vi "Certification Authority.vi"() -> ()   [LabVIEW 2013]
uses:
  certificate -- cluster.ctl
  certificate signature request (CA) -- cluster.ctl
  encryption key -- cluster.ctl
  initca -- cluster.ctl
  certificate signature request (Server) -- cluster.ctl
  <vilib>/Platform/browser.llb/Open URL in Default Browser (string).vi
  <vilib>/Platform/browser.llb/Open URL in Default Browser (path).vi
  <userlib>/_OpenG.lib/file/file.llb/Build Path - Traditional__ogtk.vi
  <userlib>/_OpenG.lib/file/file.llb/File Exists - Scalar__ogtk.vi
  <userlib>/_OpenG.lib/file/file.llb/Convert File Extension (String)__ogtk.vi
  Certification Authority.lvclass
panel:
  in  "Tab Control":T1(tab)
  in  "Root Certificate":path
  in  "Root Private Key":path
  in  "Open Certificates Folder":bool
  in  "Open GitHub Project Page":bool
  in  "Hosts":string[](array[string])=["lvtls-ca.example", "www.lvtls-ca.example"]
  in  "Common Name":string="lvtls-ca.example"
  in  "Generate Root Certificate":bool
  out "CFSSL App found":bool
  out "Root Certificate found":bool
  in  "Open Cloudflare Release Page":bool
  in  "Generate Server Certificates":bool
  in  "Servers":cluster{"hosts":string[], "name":string}[](array[cluster])
  out "Certificates":T2(array[cluster])
  in  "Certificates and Keys":i32(listbox)
  out "Selected Certificate":string
  # "ROOT (CERTIFICATE AUTHORITY)\nIf you have a root certificate and private key, import it to generate server certificate files.\nIf you don't have a root certificate, fill in the fields in section 2 and generate one."
  # "GENERATE ROOT CERTIFICATE\nIf you don't have a root certificate, fill in the fields below and generate one."
  # "3- SERVERS\nList each server you want to create certificates for."
  # "1- Give your server a unique \"Common Name\" in the name field\n2- List the hostnames that client can use to connect to this server\n     (this is not an IP address).\n3- Listing multiple servers will create certificates in batch mode.\n\n\nEx: \n\nname: myServerName\nhosts: localdomain.company.com; www.localdomain.company.com"
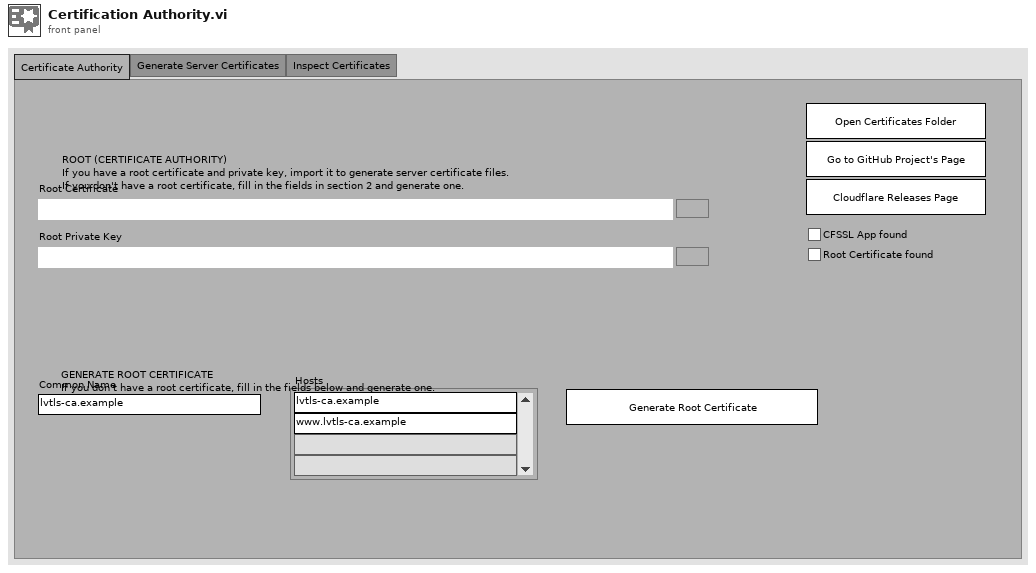
[diagram p1: front panel]
types:
  T1 = enum32{"Certificate Authority", "Generate Server Certificates", "Inspect Certificates"}
  T2 = cluster{"Type":string, "Decoded Certificate":string}[]
  T3 = enum32{"Invalid", "Standard", "Closed", "Hidden", "Minimized", "Maximized"}
  T4 = enum32{"invalid app kind", "Development System", "Run Time System", "Student Edition", "Embedded LabVIEW", "Evaluation", "Custom"}
  T5 = enum16{"open", "replace", "create", "open or create", "replace or create", "replace or create with confirmation"}
  T6 = typedef "Certification Authority.lvclass/certificate signature request (CA) -- cluster.ctl" = cluster{"CN":string, "hosts":string[], "key":T7, "ca":T8}
  T7 = typedef "Certification Authority.lvclass/encryption key -- cluster.ctl" = cluster{"algo":string, "size":u32}
  T8 = typedef "Certification Authority.lvclass/initca -- cluster.ctl" = cluster{"pathlen":u8, "expiry":string}
  T9 = typedef "Certification Authority.lvclass/certificate signature request (Server) -- cluster.ctl" = cluster{"CN":string, "hosts":string[], "key":T7}
  T10 = typedef "Certification Authority.lvclass/certificate -- cluster.ctl" = cluster{"cert":string, "csr":string, "key":string}
  T11 = cluster{"Core":cluster{"Current VI Reference":refnum<vi>, "Close Panel on Exit?":bool}, "CA":T10, "Server":T10, "cfssl path":path, "temp folder":path, "Certificates Folder":path, "Root name":string, "Root Certificate":path, "Root Private Key":path, "Active CN":string, "Active Hosts":string[], "next":i32, "Processing Queue":cluster{"hosts":string[], "name":string}[]}
  T12 = cluster{"Current VI Reference":refnum<vi>, "Close Panel on Exit?":bool}
  T13 = cluster{"Type":string, "Decoded String":string}[]
  T14 = enum8{"Enabled", "Disabled", "Disabled and Grayed Out"}
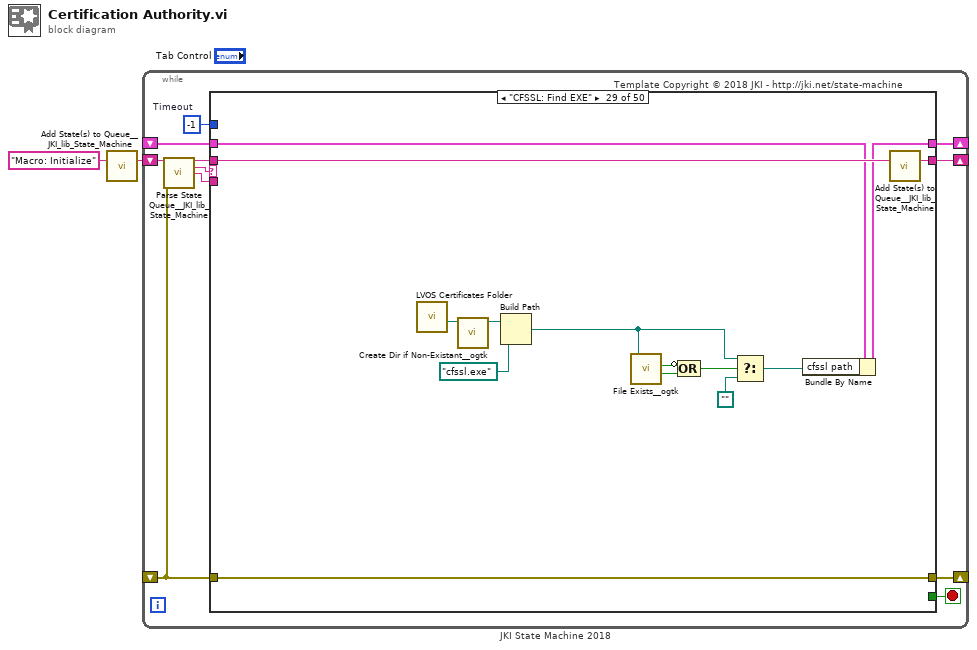
[diagram p0: block diagram]
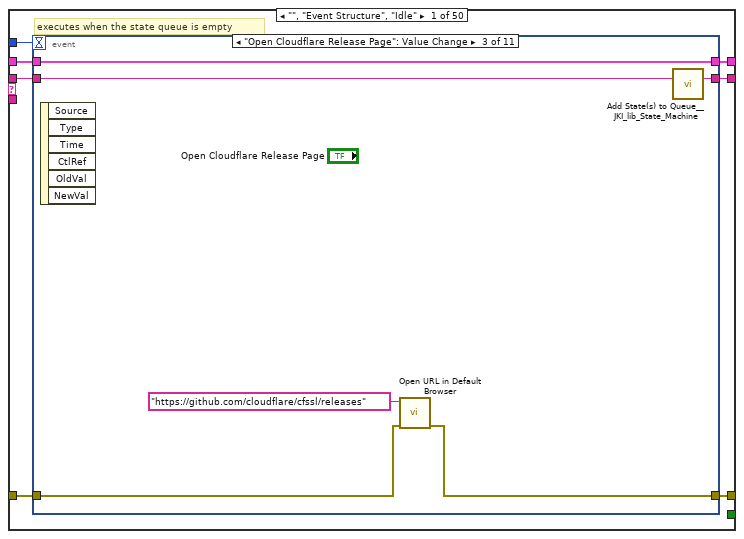
[diagram p2: hidden frame]
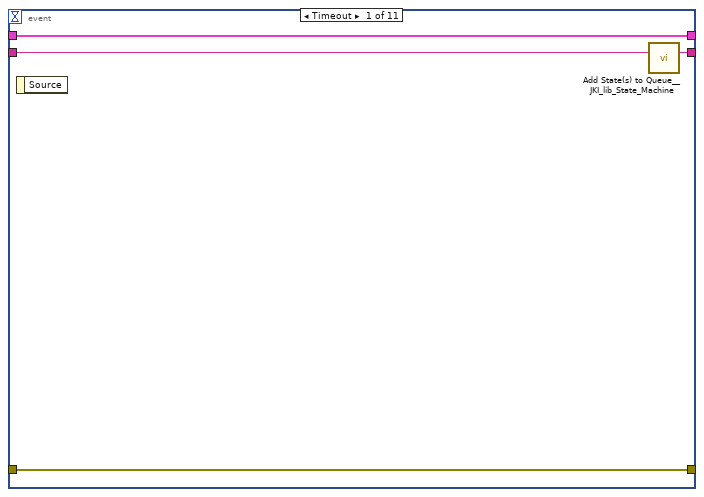
[diagram p3: hidden frame]
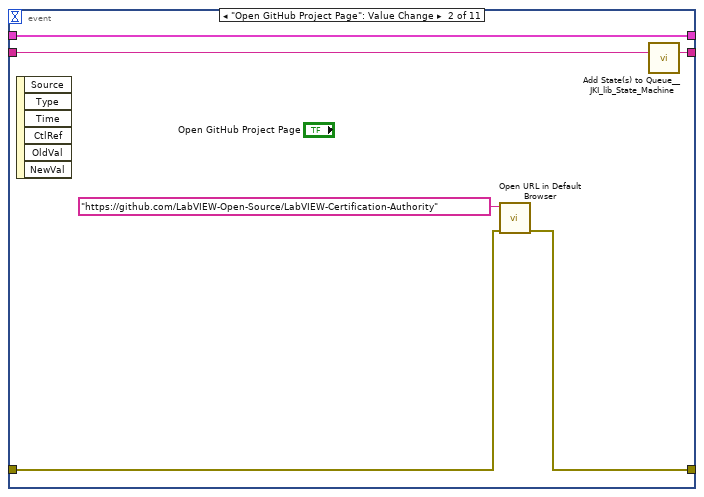
[diagram p4: hidden frame]
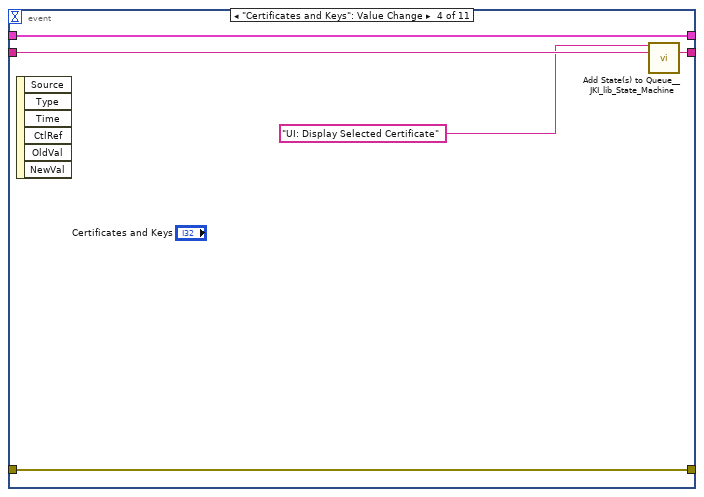
[diagram p5: hidden frame]
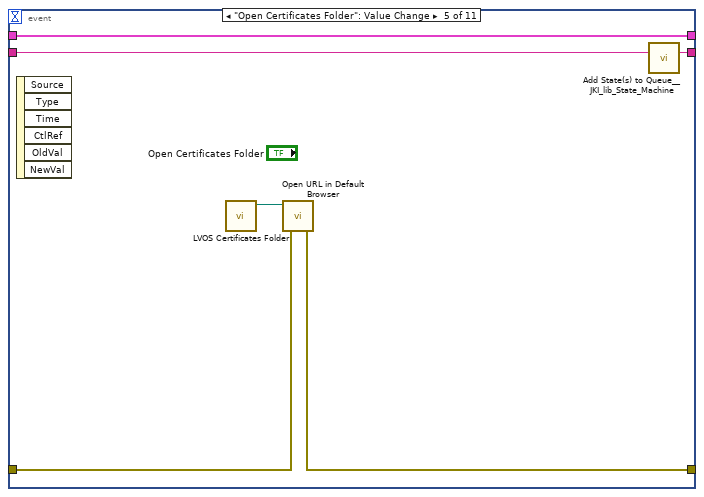
[diagram p6: hidden frame]
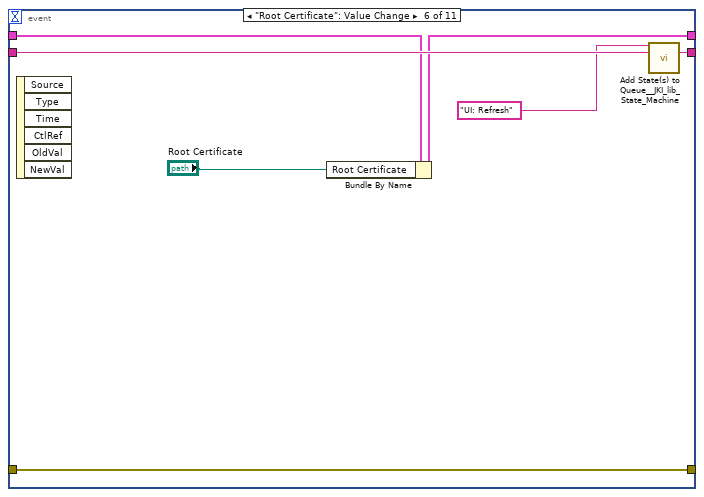
[diagram p7: hidden frame]
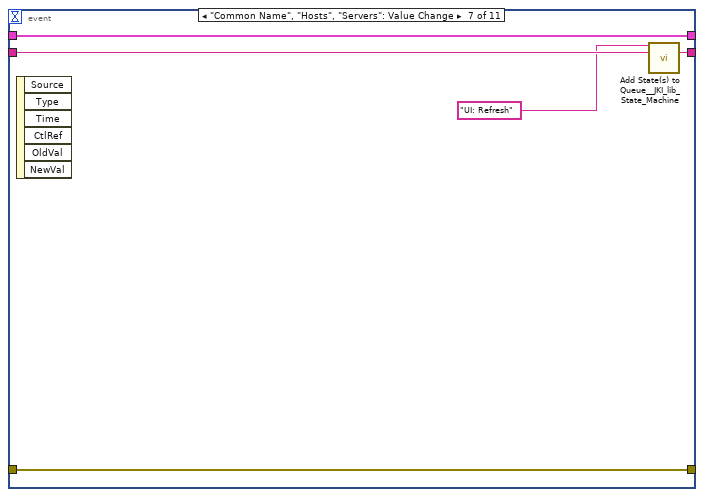
[diagram p8: hidden frame]
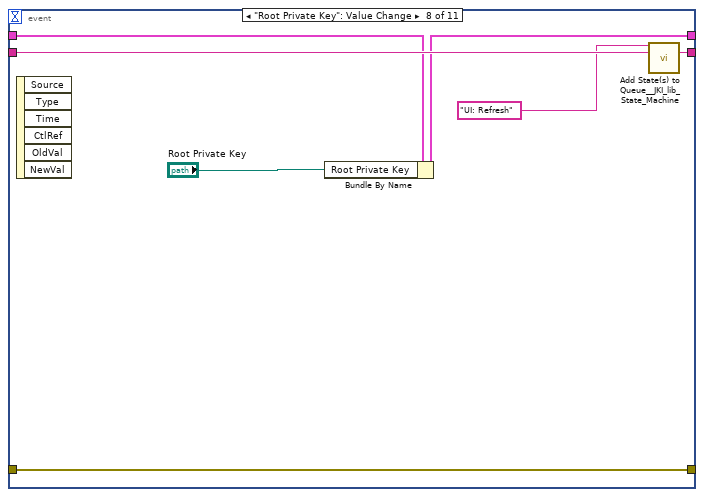
[diagram p9: hidden frame]
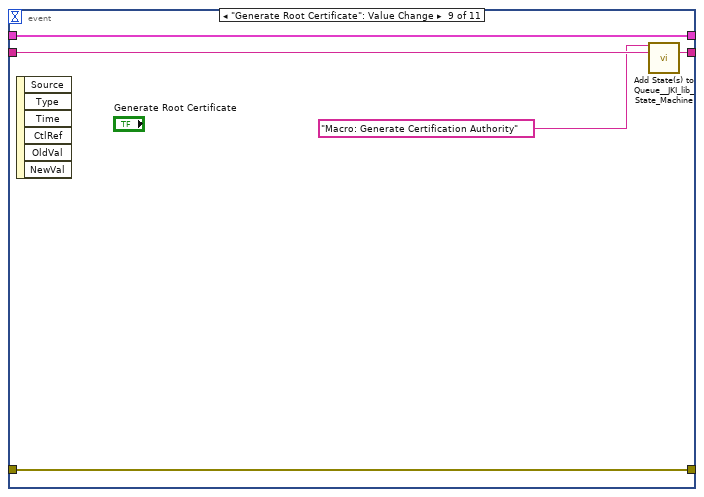
[diagram p10: hidden frame]
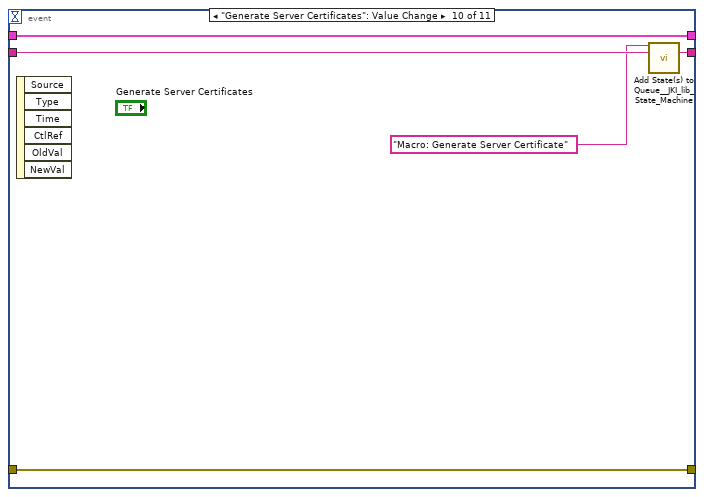
[diagram p11: hidden frame]
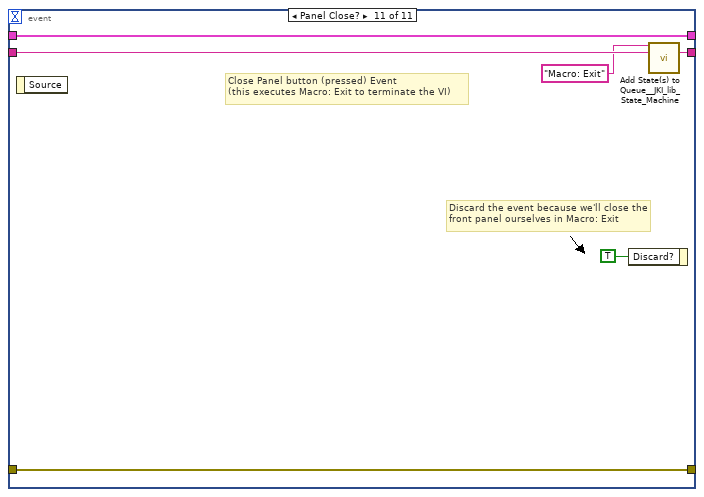
[diagram p12: hidden frame]
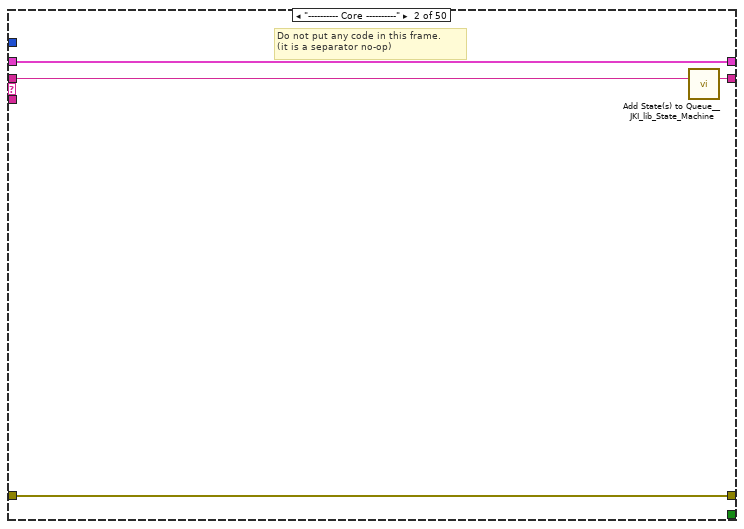
[diagram p13: hidden frame]
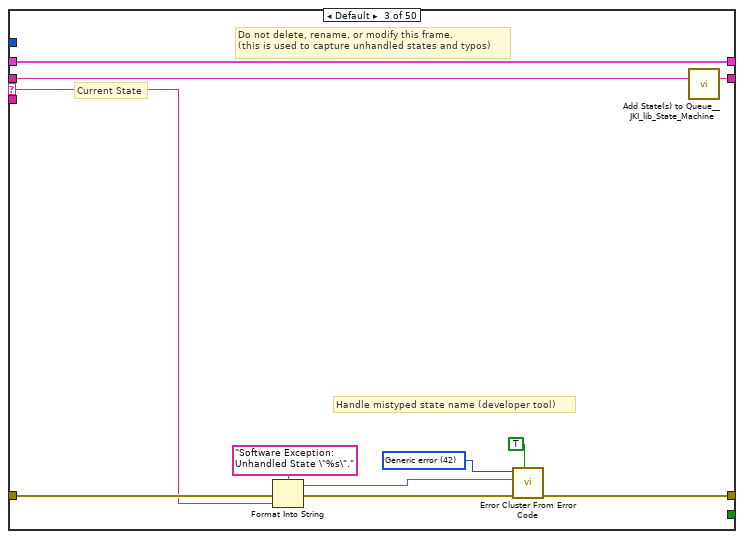
[diagram p14: hidden frame]
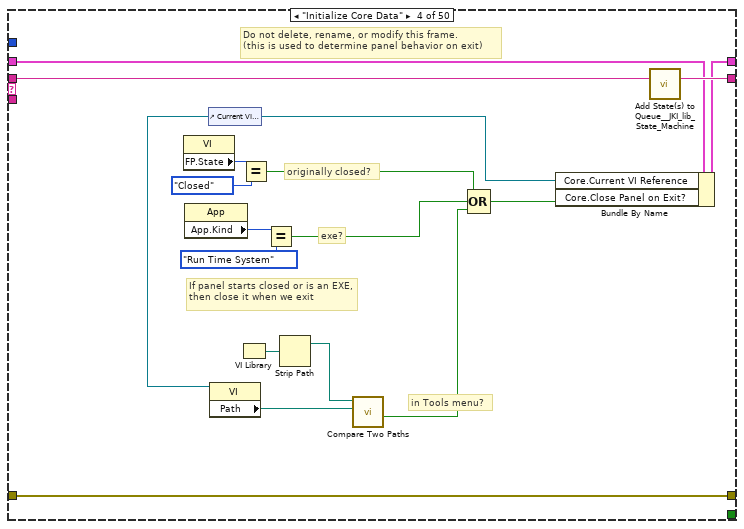
[diagram p15: hidden frame]
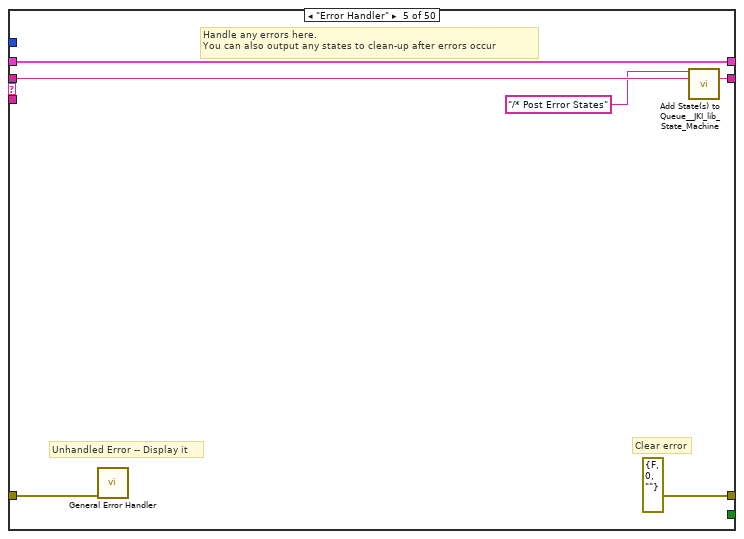
[diagram p16: hidden frame]
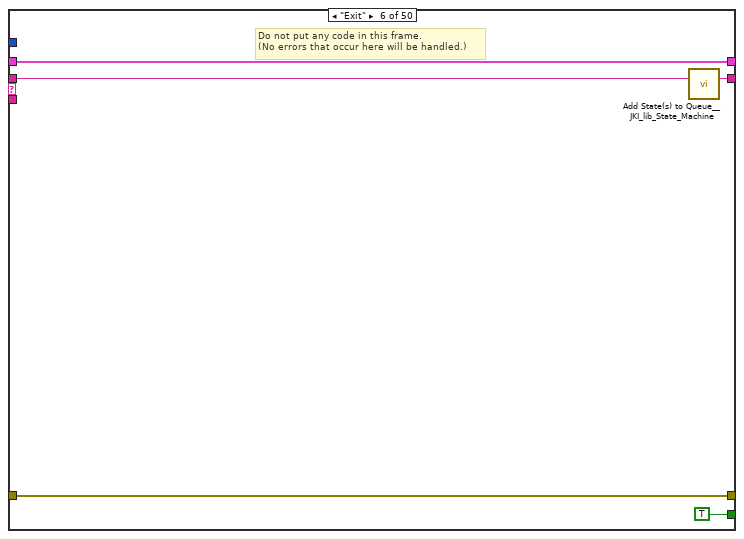
[diagram p17: hidden frame]
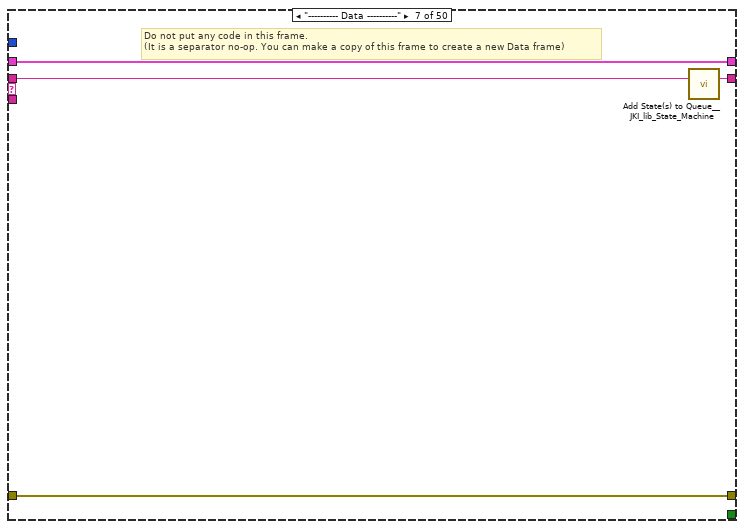
[diagram p18: hidden frame]
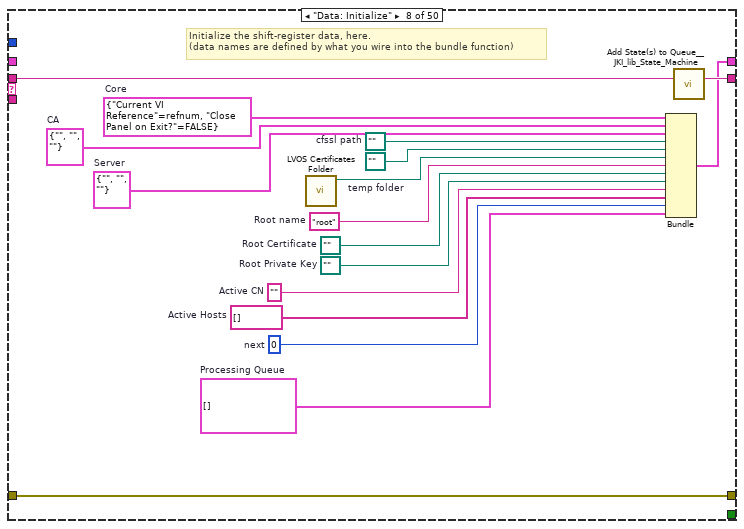
[diagram p19: hidden frame]
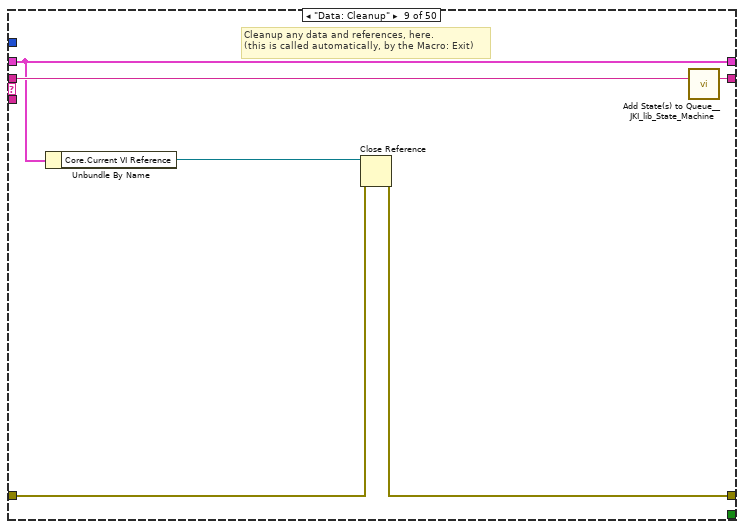
[diagram p20: hidden frame]
diagram:
  n1 = call <vilib>:"Add State(s) to Queue__JKI_lib_State_Machine.vi"("State(s) in (\"\")"="Macro: Initialize") -> ("States Out"=w2:string)  [unwired: 14 in]
  n2 = while "JKI State Machine 2018" {
    shift-right: [w6] -> _
    shift-left: _ -> [w5]
    shift-right: [w9] -> _
    shift-left: _ -> [w3]
    shift-right: [w8] -> _
    shift-left: w2 -> [w10]
    stop <- w7 stop-if-true
    w4 = -1  # Timeout
    # "Template Copyright © 2018 JKI - http://jki.net/state-machine"
    n3 = call <vilib>:"Parse State Queue__JKI_lib_State_Machine.vi"("State Queue"=w10, "Error In (no error)"=w3) -> ("Remaining States"=w12:string, "Current State"=w13:string, "Arguments"=w11:string)  [unwired: 11 in]
    n4 = case shown="\"CFSSL: Find EXE\"" w13 {
      selector: w13 -> [_ _ w87 _ _ _ _ _ _ _ _ _ _ _ _ _ _ _ _ _ _ _ _ _ _ _ _ _ _ _ _ _ _ _ _ _ _ _ _ _ _ _ _ _ _ _ _ _ _ _]
      tunnel: w12 -> [w20 w86 w91 w114 w120 w125 w129 w146 w152 w156 w165 w176 w185 w240 w244 w248 w253 w259 w270 w339 w344 w349 w357 w362 w371 w376 w387 w391 w405 w414 w424 w451 w466 w481 w504 w525 w542 w552 w566 w597 w620 w646 w669 w701 w718 w735 w752 w769 w786 w803]
      tunnel: w11 -> [_ _ _ _ _ _ _ _ _ _ _ _ _ _ _ _ _ w254 w264 _ _ _ _ _ _ _ _ _ _ _ _ _ _ _ _ _ _ _ _ _ _ _ _ _ _ _ _ _ _ _]
      tunnel: w5 -> [w18 w83 w89 w107 w117 w123 w126 _ w147 w153 w163 w174 w183 w210 w241 w245 w250 w257 w266 w336 w341 w346 w353 w359 w368 w373 w384 w388 w402 w412 w422 w447 w455 w471 w502 w523 w535 w547 w564 w567 w613 w642 w659 w684 w710 w727 w744 w761 w778 w795]
      tunnel: [w17 w84 w93 w111 errorcluster {"status"=FALSE, "code"=0, "source"=""} ("error out") w122 w127 w143 w148 w154 w159 w171 w180 w238 w242 w246 w251 w255 w267 w337 w342 w347 w355 w360 w369 w374 w385 w389 w403 w407 w418 w449 w452 w468 w482 w511 w528 w543 w555 w570 w615 w643 w648 w685 w705 w722 w739 w756 w773 w790] -> w9
      tunnel: w3 -> [w16 w84 w92 w111 w116 w122 w127 w143 w149 w154 w160 w172 w180 w238 w242 w246 w251 w256 w268 w337 w342 w347 w355 w360 w369 w374 w385 w389 w403 w408 w417 w449 w453 w469 w483 w512 w529 w543 w553 w574 w616 w644 w651 w688 w707 w724 w741 w758 w775 w792]
      tunnel: [w19 w85 w90 w113 w119 w124 w128 w145 w151 w155 w164 w175 w184 w239 w243 w247 w252 w258 w269 w338 w343 w348 w356 w361 w370 w375 w386 w390 w404 w413 w423 w450 w465 w480 w503 w524 w541 w551 w565 w596 w619 w645 w668 w700 w717 w734 w751 w768 w785 w802] -> w8
      tunnel: [_ _ _ _ _ TRUE _ _ _ _ _ _ _ _ _ _ _ _ _ _ _ _ _ _ _ _ _ _ _ _ _ _ _ _ _ _ _ _ _ _ _ _ _ _ _ _ _ _ _ _] -> w7
      tunnel: [w15 w83 w89 w112 w117 w123 w126 w144 w147 w153 w163 w174 w183 w210 w241 w245 w250 w257 w266 w336 w341 w346 w352 w359 w368 w373 w384 w388 w401 w411 w422 w448 w456 w472 w502 w523 w535 w550 w564 w567 w612 w641 w659 w684 w710 w727 w744 w761 w778 w795] -> w6
      tunnel: w4 -> [w14 _ _ _ _ _ _ _ _ _ _ _ _ _ _ _ _ _ _ _ _ _ _ _ _ _ _ _ _ _ _ _ _ _ _ _ _ _ _ _ _ _ _ _ _ _ _ _ _ _]
      frame "", "Event Structure", "Idle" {
        # "executes when the state queue is empty"
        n5 = event shown="[2] \"Open Cloudflare Release Page\": Value Change" {
          selector: _ -> [_ _ _ _ _ _ _ _ _ _ _]
          dyn-events: _ -> [_ _ _ _ _ _ _ _ _ _ _]
          timeout: w14 -> [_ _ _ _ _ _ _ _ _ _ _]
          tunnel: w20 -> [w24 w30 w36 w41 w47 w54 w59 w66 w71 w76 w82]
          tunnel: [w23 w29 w35 w40 w46 w53 w58 w65 w70 w75 w81] -> w19
          tunnel: w18 -> [w21 w28 w34 w38 w45 w51 w55 w63 w68 w73 w79]
          tunnel: [w22 w25 w31 w39 w42 w52 w57 w64 w69 w74 w80] -> w17
          tunnel: w16 -> [w22 w26 w32 w39 w43 w52 w57 w64 w69 w74 w80]
          tunnel: [w21 w28 w34 w38 w45 w50 w55 w62 w68 w73 w79] -> w15
          event Timeout {
            n6 = event-data() -> ()  [unwired: 1 in, 1 out]
            n7 = call <vilib>:"Add State(s) to Queue__JKI_lib_State_Machine.vi"("State(s) in (\"\")"=w24) -> ("States Out"=w23:string)  [unwired: 14 in]
          }
          event "Open GitHub Project Page": Value Change {
            n8 = event-data() -> ()  [unwired: 1 in, 6 out]
            n9 = call-poly <vilib>:"Open URL in Default Browser.vi"("error in (no error)"=w26, "URL"="https://github.com/LabVIEW-Open-Source/LabVIEW-Certification-Authority") -> ("error out"=w25:errorcluster)  [unwired: 4 in, 1 out]
            n10 = call <vilib>:"Add State(s) to Queue__JKI_lib_State_Machine.vi"("State(s) in (\"\")"=w30) -> ("States Out"=w29:string)  [unwired: 14 in]
          }
          event "Open Cloudflare Release Page": Value Change {
            n11 = event-data() -> ()  [unwired: 1 in, 6 out]
            n12 = call-poly <vilib>:"Open URL in Default Browser.vi"("error in (no error)"=w32, "URL"="https://github.com/cloudflare/cfssl/releases") -> ("error out"=w31:errorcluster)  [unwired: 4 in, 1 out]
            n13 = call <vilib>:"Add State(s) to Queue__JKI_lib_State_Machine.vi"("State(s) in (\"\")"=w36) -> ("States Out"=w35:string)  [unwired: 14 in]
          }
          event "Certificates and Keys": Value Change {
            n14 = event-data() -> ()  [unwired: 1 in, 6 out]
            n15 = call <vilib>:"Add State(s) to Queue__JKI_lib_State_Machine.vi"("State(s) in Front (\"\")"="UI: Display Selected Certificate", "State(s) in (\"\")"=w41) -> ("States Out"=w40:string)  [unwired: 13 in]
          }
          event "Open Certificates Folder": Value Change {
            n16 = event-data() -> ()  [unwired: 1 in, 6 out]
            n17 = call "LVOS Certificates Folder.vi"() -> ("Certificates Folder"=w44:path)  [unwired: 10 in, 1 out]
            n18 = call-poly <vilib>:"Open URL in Default Browser.vi"("error in (no error)"=w43, "path"=w44) -> ("error out"=w42:errorcluster)  [unwired: 4 in, 1 out]
            n19 = call <vilib>:"Add State(s) to Queue__JKI_lib_State_Machine.vi"("State(s) in (\"\")"=w47) -> ("States Out"=w46:string)  [unwired: 14 in]
          }
          event "Root Certificate": Value Change {
            n20 = event-data() -> ()  [unwired: 1 in, 6 out]
            n21 = Bundle By Name(cluster=w51, "Root Certificate"="Root Certificate") -> (w50:T11)
            n22 = call <vilib>:"Add State(s) to Queue__JKI_lib_State_Machine.vi"("State(s) in Front (\"\")"="UI: Refresh", "State(s) in (\"\")"=w54) -> ("States Out"=w53:string)  [unwired: 13 in]
          }
          event "Common Name", "Hosts", "Servers": Value Change {
            n23 = event-data() -> ()  [unwired: 1 in, 6 out]
            n24 = call <vilib>:"Add State(s) to Queue__JKI_lib_State_Machine.vi"("State(s) in Front (\"\")"="UI: Refresh", "State(s) in (\"\")"=w59) -> ("States Out"=w58:string)  [unwired: 13 in]
          }
          event "Root Private Key": Value Change {
            n25 = event-data() -> ()  [unwired: 1 in, 6 out]
            n26 = Bundle By Name(cluster=w63, "Root Private Key"="Root Private Key") -> (w62:T11)
            n27 = call <vilib>:"Add State(s) to Queue__JKI_lib_State_Machine.vi"("State(s) in Front (\"\")"="UI: Refresh", "State(s) in (\"\")"=w66) -> ("States Out"=w65:string)  [unwired: 13 in]
          }
          event "Generate Root Certificate": Value Change {
            n28 = event-data() -> ()  [unwired: 1 in, 6 out]
            n29 = call <vilib>:"Add State(s) to Queue__JKI_lib_State_Machine.vi"("State(s) in Front (\"\")"="Macro: Generate Certification Authority", "State(s) in (\"\")"=w71) -> ("States Out"=w70:string)  [unwired: 13 in]
          }
          event "Generate Server Certificates": Value Change {
            n30 = event-data() -> ()  [unwired: 1 in, 6 out]
            n31 = call <vilib>:"Add State(s) to Queue__JKI_lib_State_Machine.vi"("State(s) in Front (\"\")"="Macro: Generate Server Certificate", "State(s) in (\"\")"=w76) -> ("States Out"=w75:string)  [unwired: 13 in]
          }
          event Panel Close? {
            # "Discard the event because we'll close the front panel ourselves in Macro: Exit"
            # "Close Panel button (pressed) Event\n(this executes Macro: Exit to terminate the VI)"
            n32 = event-data() -> ()  [unwired: 1 in, 1 out]
            n33 = event-data("Discard?"=TRUE) -> ()  [unwired: 1 in, 1 out]
            n34 = call <vilib>:"Add State(s) to Queue__JKI_lib_State_Machine.vi"("State(s) in Front (\"\")"="Macro: Exit", "State(s) in (\"\")"=w82) -> ("States Out"=w81:string)  [unwired: 13 in]
          }
        }
      }
      frame "---------- Core ----------" {
        # "Do not put any code in this frame.\n(it is a separator no-op)"
        n35 = call <vilib>:"Add State(s) to Queue__JKI_lib_State_Machine.vi"("State(s) in (\"\")"=w86) -> ("States Out"=w85:string)  [unwired: 14 in]
      }
      frame Default {
        w96 = 42 items=["No error", "Argument error", "Memory is full", "Out of zone", "End of file", "File already open", "Generic file I/O error", "File not found", "File permission error", "Disk is full", "Duplicate path", "Too many files open", "System feature not enabled", "Resource file not found", "Cannot add resource", "Resource not found", "Image not found", "Image memory error", "Pen does not exist", "Config type invalid", "Config token not found", "Config parse error", "Config memory error", "Bad external code format", "Bad external code offset", "External code not present", "Null window", "Destroy window error", "Null menu", "Print aborted", "Bad print record", "Print driver error", "Windows error during printing", "Memory error during printing", "Print dialog error", "Generic print error", "Invalid device refnum", "Device not found", "Device parameter error", "Device unit error", "Cannot open device", "Device call aborted", "Generic error", "Cancelled by user", "Object ID too low", "Object ID too high", "Object not in heap", "Unknown heap", "Unknown object (invalid DefProc)", "Unknown object (DefProc not in table)", "Message out of range", "Invalid (null) method", "Unknown message", "Manager call not supported", "Bad address", "Network operation in progress", "Network operation timed out", "Connection is busy", "Network attribute not supported", "Network error", "Address in use", "System out of memory", "Connection aborted", "Connection refused", "Not connected", "Already connected", "Connection closed", "Initialization error (interapplication manager)", "Bad occurrence", "Wait on unbound occurrence handler", "Occurrence queue overflow", "Datalog type conflict", "Unused", "Unrecognized type (interapplication manager)", "Memory corrupt", "Failed to make temporary DLL", "Old CIN version", "Drag socket not found", "Failed to load drop-object", "Failed to register OLE object", "Failed to release OLE object", "Format specifier type mismatch", "Unknown format specifier", "Too few format specifiers", "Too many format specifiers", "Scan failed", "Newer CIN version", "Error converting to variant", "Runtime menu error", "Password tampered", "Variant attribute not found", "Incompatible variant data type", "Event data is not available", "Event Store is not present", "Occurrence is not found", "Event Queue is not created", "Event info is not available", "Refnum passed is NULL", "Error retrieving Class GUID", "Error retrieving CoClass GUID", "Error retrieving TypeLib GUID.", "Bad built application magic bytes.", "Specific driver is different from the specific driver associated with the Logical Name.", "There is no session opened to the class driver.", "Max Error", "MAX - Error with config objects", "MAX - Error loading configuration", "MAX - Group not supported"]
        # "Current State"
        # "Do not delete, rename, or modify this frame.\n(this is used to capture unhandled states and typos)"
        # "Handle mistyped state name (developer tool)"
        n36 = Format Into String(format string="Software Exception: Unhandled State \"%s\"." ("message"), error in=w92, w87) -> (resulting string=w95:string, error out=w94:errorcluster)  [unwired: 1 in]
        n37 = call <vilib>:"Error Cluster From Error Code.vi"("show call chain? (False)"=TRUE, "error in (no error)"=w94, "error message (\"\")"=w95, "error code (0)"=w96) -> ("error out"=w93:errorcluster)  [unwired: 5 in]
        n38 = call <vilib>:"Add State(s) to Queue__JKI_lib_State_Machine.vi"("State(s) in (\"\")"=w91) -> ("States Out"=w90:string)  [unwired: 14 in]
      }
      frame "Initialize Core Data" {
        # "in Tools menu?"
        # "Do not delete, rename, or modify this frame.\n(this is used to determine panel behavior on exit)"
        # "originally closed?"
        # "exe?"
        # "If panel starts closed or is an EXE, then close it when we exit"
        n39 = property class="VI"() -> ("FP.State"=w105:T3)  [unwired: 2 in, 2 out]
        n40 = property class="App"() -> ("App.Kind"=w110:T4)  [unwired: 2 in, 2 out]
        n41 = control-ref of="Current VI Reference"() -> (w102:refnum<vi>)
        n42 = property class="VI"(reference=w102) -> ("Path"=w101:path)  [unwired: 1 in, 2 out]
        n43 = VI Library() -> (path=w100:path)
        n44 = Equal?(x=w105, y=T3."Closed" ("Front Panel Window:State")) -> (x = y?=w103:bool)
        n45 = Equal?(x=w110, y=T4."Run Time System" ("Application:Kind")) -> (x = y?=w108:bool)
        n46 = Strip Path(path=w100) -> (stripped path=w99:path)  [unwired: 1 out]
        n47 = call <vilib>:"Compare Two Paths.vi"("Path 2"=w101, "Path 1"=w99) -> ("Path 2 Relative to Path 1?"=w98:bool)  [unwired: 6 in, 3 out]
        n48 = Compound Arithmetic op=OR(w103, w108, w98) -> (w106:bool)
        n49 = Bundle By Name(cluster=w107, "Core.Current VI Reference"=w102, "Core.Close Panel on Exit?"=w106) -> (w112:T11)
        n50 = call <vilib>:"Add State(s) to Queue__JKI_lib_State_Machine.vi"("State(s) in (\"\")"=w114) -> ("States Out"=w113:string)  [unwired: 14 in]
      }
      frame "Error Handler" {
        # "Unhandled Error -- Display it"
        # "Handle any errors here.\nYou can also output any states to clean-up after errors occur"
        # "Clear error"
        n51 = call <vilib>:"General Error Handler.vi"("error in (no error)"=w116) -> ()  [unwired: 10 in, 5 out]
        n52 = call <vilib>:"Add State(s) to Queue__JKI_lib_State_Machine.vi"("State(s) in Front (\"\")"="/* Post Error States", "State(s) in (\"\")"=w120) -> ("States Out"=w119:string)  [unwired: 13 in]
      }
      frame "Exit" {
        # "Do not put any code in this frame.\n(No errors that occur here will be handled.)"
        n53 = call <vilib>:"Add State(s) to Queue__JKI_lib_State_Machine.vi"("State(s) in (\"\")"=w125) -> ("States Out"=w124:string)  [unwired: 14 in]
      }
      frame "---------- Data ----------" {
        # "Do not put any code in this frame.\n(It is a separator no-op. You can make a copy of this frame to create a new Data frame)"
        n54 = call <vilib>:"Add State(s) to Queue__JKI_lib_State_Machine.vi"("State(s) in (\"\")"=w129) -> ("States Out"=w128:string)  [unwired: 14 in]
      }
      frame "Data: Initialize" {
        w130 = cluster{"hosts":string[], "name":string}[] []  # Processing Queue
        w131 = 0  # next
        w133 = string[] []  # Active Hosts
        w134 = ""  # Active CN
        w135 = path ""  # Root Private Key
        w136 = path ""  # Root Certificate
        w137 = "root"  # Root name
        w138 = path ""  # temp folder
        w139 = path ""  # cfssl path
        w140 = T10 {"cert"="", "csr"="", "key"=""}  # Server
        w141 = T10 {"cert"="", "csr"="", "key"=""}  # CA
        w142 = T12 {"Current VI Reference"=refnum, "Close Panel on Exit?"=FALSE}  # Core
        # "Initialize the shift-register data, here.\n(data names are defined by what you wire into the bundle function)"
        n55 = call "LVOS Certificates Folder.vi"() -> ("Certificates Folder"=w132:path)  [unwired: 10 in, 1 out]
        n56 = Bundle("Core"=w142, "CA"=w141, "Server"=w140, "cfssl path"=w139, "temp folder"=w138, "Certificates Folder"=w132, "Root name"=w137, "Root Certificate"=w136, "Root Private Key"=w135, "Active CN"=w134, "Active Hosts"=w133, "next"=w131, "Processing Queue"=w130) -> (w144:T11)  [unwired: 1 in]
        n57 = call <vilib>:"Add State(s) to Queue__JKI_lib_State_Machine.vi"("State(s) in (\"\")"=w146) -> ("States Out"=w145:string)  [unwired: 14 in]
      }
      frame "Data: Cleanup" {
        # "Cleanup any data and references, here.\n(this is called automatically, by the Macro: Exit)"
        n58 = Unbundle By Name(w147) -> ("Core.Current VI Reference"=w150:refnum<vi>)
        n59 = Close Reference(reference=w150, error in (no error)=w149) -> (error out=w148:errorcluster)
        n60 = call <vilib>:"Add State(s) to Queue__JKI_lib_State_Machine.vi"("State(s) in (\"\")"=w152) -> ("States Out"=w151:string)  [unwired: 14 in]
      }
      frame "---------- UI ----------" {
        # "Do not put any code in this frame.\n(It is a separator no-op. You can make a copy of this frame to create a new UI frame)"
        n61 = call <vilib>:"Add State(s) to Queue__JKI_lib_State_Machine.vi"("State(s) in (\"\")"=w156) -> ("States Out"=w155:string)  [unwired: 14 in]
      }
      frame "UI: Initialize" {
        # "Initialize the User Interface, here.\n(this is called automatically, by the Macro: Init)"
        n62 = property on="Certificates and Keys" class="LstBox (strict)"("Item Names"=string[] []) -> ()  [unwired: 2 in, 2 out]
        n63 = local write "Tab Control"(0) -> ()
        n64 = call "LVOS Certificates Folder.vi"() -> ("Certificates Folder"=w162:path)  [unwired: 10 in, 1 out]
        n65 = call <userlib>:"Create Dir if Non-Existant__ogtk.vi"("error in (no error)"=w160, "Directory Path"=w162) -> ("error out"=w159:errorcluster, "dup Directory Path"=w161:path)  [unwired: 7 in, 1 out]
        n66 = invoke on="Servers" class="Arr (strict)" method="Reinit To Default"() -> ()  [unwired: 3 in, 3 out]
        n67 = property on="Root Private Key" class="Path"("StartPath"=w161) -> ()  [unwired: 2 in, 2 out]
        n68 = property on="Root Certificate" class="Path"("StartPath"=w161) -> ()  [unwired: 2 in, 2 out]
        n69 = call <vilib>:"Add State(s) to Queue__JKI_lib_State_Machine.vi"("State(s) in (\"\")"=w165) -> ("States Out"=w164:string)  [unwired: 14 in]
      }
      frame "UI: List Certificates" {
        n70 = call "LVOS Certificates Folder.vi"() -> ("Certificates Folder"=w173:path)  [unwired: 10 in, 1 out]
        n71 = call <userlib>:"Create Dir if Non-Existant__ogtk.vi"("error in (no error)"=w172, "Directory Path"=w173) -> ("error out"=w171:errorcluster, "dup Directory Path"=w170:path)  [unwired: 7 in, 1 out]
        n72 = call <userlib>:"List Directory__ogtk.vi"("pattern"="*.pem; *.crt; *.csr", "directory path"=w170) -> ("file names"=w168:string[])  [unwired: 2 in, 3 out]
        n73 = Sort 1D Array(array=w168) -> (sorted array=w167:string[])
        n74 = property on="Certificates and Keys" class="LstBox (strict)"("Item Names"=w167, "Value"=-1 ("Trusted Certificates")) -> ()  [unwired: 2 in, 2 out]
        n75 = call <vilib>:"Add State(s) to Queue__JKI_lib_State_Machine.vi"("State(s) in (\"\")"=w176) -> ("States Out"=w175:string)  [unwired: 14 in]
      }
      frame "UI: Display Selected Certificate" {
        n76 = property on="Certificates and Keys" class="LstBox (strict)"() -> ("Item Names"=w182:string[], "Value"=w181:i32)  [unwired: 2 in, 2 out]
        n77 = Index Array(array=w182, index=w181) -> (element=w179:string)
        n78 = case shown="Default" w179 {
          selector: w179 -> [w192 _]
          tunnel: [w186 _] -> w178
          frame Default {
            n79 = call "LVOS Certificates Folder.vi"() -> ("Certificates Folder"=w193:path)  [unwired: 10 in, 1 out]
            n80 = call-poly <userlib>:"Build Path__ogtk.vi"("name or relative path"=w192, "base path"=w193) -> ("appended path"=w188:path)
            n81 = call-poly <userlib>:"File Exists__ogtk.vi"("file path"=w188) -> ("is directory"=w191:bool, "exists"=w190:bool)  [unwired: 6 in]
            n82 = Empty String/Path?(string/path=w188) -> (empty?=w189:bool)
            n83 = Compound Arithmetic op=AND(invert w191, w190, invert w189) -> (w187:bool)
            n84 = case shown="True" w187 {
              tunnel: w188 -> [_ w195]
              tunnel: [_ w194] -> w186
              frame False {
              }
              frame True {
                n85 = Open/Create/Replace File(file path (use dialog)=w195, operation (0:open)=T5."open", access (0:read/write)=enum16{"read/write", "read-only", "write-only"}."read-only") -> (refnum out=w200:refnum<file>, error out=w201:errorcluster)  [unwired: 3 in, 1 out]
                n86 = Read from Text File(file (use dialog)=w200, error in=w201) -> (refnum out=w198:refnum<file>, text=w194:string, error out=w199:errorcluster)  [unwired: 2 in, 1 out]
                n87 = Close File(refnum=w198, error in=w199) -> ()  [unwired: 2 out]
              }
            }
          }
          frame "" {
          }
        }
        "Selected Certificate" <- w178
        n88 = call "Inspect Certificate.vi"("Certificate string"=w178) -> ("Certificates"=→"Certificates":T13)  [unwired: 10 in]
        n89 = call <vilib>:"Add State(s) to Queue__JKI_lib_State_Machine.vi"("State(s) in (\"\")"=w185) -> ("States Out"=w184:string)  [unwired: 14 in]
      }
      frame "UI: Refresh" {
        w215 = T14."Disabled and Grayed Out" ("Disabled")
        w214 = T14."Enabled" ("Disabled")
        n90 = Unbundle By Name(w210) -> ("Certificates Folder"=w235:path)
        n91 = Unbundle By Name(w210) -> ("Root Certificate"=w212:path, "Root Private Key"=w211:path)
        n92 = local read "Common Name"() -> (w219:string)
        n93 = local read "Servers"() -> (w232:cluster{"hosts":string[], "name":string}[])
        n94 = Unbundle By Name(w210) -> ("cfssl path"=w209:path)
        n95 = local read "Hosts"() -> (w218:string[])
        n96 = Not A Number/Path/Refnum?(number/path/refnum=w209) -> (NaN/Path/Refnum?=w204:bool)
        n97 = local write "Root Private Key"(w211) -> ()
        n98 = call-poly <userlib>:"File Exists__ogtk.vi"("file path"=w235) -> ("is directory"=w233:bool, "exists"=w234:bool)  [unwired: 6 in]
        n99 = Empty String/Path?(string/path=w235) -> (empty?=w236:bool)
        n100 = Empty Array?(array=w232) -> (empty?=w237:bool)
        n101 = Empty String/Path?(string/path=w219) -> (empty?=w217:bool)
        n102 = local write "Root Certificate"(w212) -> ()
        n103 = call-poly <userlib>:"File Exists__ogtk.vi"("file path"=w212) -> ("is directory"=w229:bool, "exists"=w228:bool)  [unwired: 6 in]
        n104 = call-poly <userlib>:"File Exists__ogtk.vi"("file path"=w211) -> ("is directory"=w224:bool, "exists"=w225:bool)  [unwired: 6 in]
        n105 = Empty String/Path?(string/path=w212) -> (empty?=w227:bool)
        n106 = Empty String/Path?(string/path=w211) -> (empty?=w226:bool)
        n107 = Empty Array?(array=w218) -> (empty?=w216:bool)
        n108 = Compound Arithmetic op=AND(invert w229, w228, invert w227) -> (w223:bool)
        n109 = Compound Arithmetic op=AND(invert w224, w225, invert w226) -> (w222:bool)
        n110 = Compound Arithmetic op=AND(w223, w222) -> (w202:bool)
        "Root Certificate found" <- w202
        n111 = Not(x=w204) -> (.not. x?=→"CFSSL App found":bool)
        n112 = Not(x=w202) -> (.not. x?=w206:bool)
        n113 = Compound Arithmetic op=AND(w206, invert w204) -> (w207:bool)
        n114 = Compound Arithmetic op=AND(w202, w233, w234, invert w236, invert w237, invert w204) -> (w230:bool)
        n115 = Compound Arithmetic op=AND(w206, invert w204) -> (w205:bool)
        n116 = Compound Arithmetic op=AND(invert w217, invert w216, w206, invert w204) -> (w208:bool)
        n117 = Select(t=w214, s=w205, f=w215) -> (s? t:f=w220:T14)
        n118 = Select(t=w214, s=w207, f=w215) -> (s? t:f=w221:T14)
        n119 = Select(t=w214, s=w208, f=w215) -> (s? t:f=w213:T14)
        n120 = Select(t=w214, s=w230, f=w215) -> (s? t:f=w231:T14)
        n121 = property on="Generate Root Certificate" class="Bool"("DisabledEnum"=w213) -> ()  [unwired: 2 in, 2 out]
        n122 = property on="Generate Server Certificates" class="Bool"("DisabledEnum"=w231) -> ()  [unwired: 2 in, 2 out]
        n123 = property on="Common Name" class="Str"("DisabledEnum"=w220) -> ()  [unwired: 2 in, 2 out]
        n124 = property on="hostname" class="Str"("DisabledEnum"=w221) -> ()  [unwired: 2 in, 2 out]
        n125 = call <vilib>:"Add State(s) to Queue__JKI_lib_State_Machine.vi"("State(s) in (\"\")"=w240) -> ("States Out"=w239:string)  [unwired: 14 in]
      }
      frame "UI: Display CA" {
        n126 = Unbundle By Name(w241) -> ()  [unwired: 1 out]
        n127 = call <vilib>:"Add State(s) to Queue__JKI_lib_State_Machine.vi"("State(s) in (\"\")"=w244) -> ("States Out"=w243:string)  [unwired: 14 in]
      }
      frame "UI: Display Server Cert" {
        n128 = Unbundle By Name(w245) -> ()  [unwired: 1 out]
        n129 = call <vilib>:"Add State(s) to Queue__JKI_lib_State_Machine.vi"("State(s) in (\"\")"=w248) -> ("States Out"=w247:string)  [unwired: 14 in]
      }
      frame "UI: Show Temporary Folder" {
        n130 = Unbundle By Name(w250) -> ("temp folder"=w249:path)
        n131 = call-poly <vilib>:"Open URL in Default Browser.vi"("path"=w249) -> ()  [unwired: 5 in, 2 out]
        n132 = call <vilib>:"Add State(s) to Queue__JKI_lib_State_Machine.vi"("State(s) in (\"\")"=w253) -> ("States Out"=w252:string)  [unwired: 14 in]
      }
      frame "UI: Cursor Set" {
        # "Argument"
        # "Set and Unset Cursor Busy.\n(Usage: \"UI: Cursor Set >> Busy|Idle\")"
        n133 = case shown="\"Idle\", Default" w254 {
          tunnel: w256 -> [w261 w263]
          tunnel: [w260 w262] -> w255
          frame "Idle", Default {
            n134 = call <vilib>:"Unset Busy.vi"("error in (no error)"=w261) -> ("error out"=w260:errorcluster)  [unwired: 10 in]
          }
          frame "Busy" {
            n135 = call <vilib>:"Set Busy.vi"("error in (no error)"=w263) -> ("error out"=w262:errorcluster)  [unwired: 9 in, 1 out]
          }
        }
        n136 = call <vilib>:"Add State(s) to Queue__JKI_lib_State_Machine.vi"("State(s) in (\"\")"=w259) -> ("States Out"=w258:string)  [unwired: 14 in]
      }
      frame "UI: Front Panel State" {
        # "Argument"
        # "Set Front Panel Open or Closed\n(Usage: \"UI: Front Panel State >> Open|Close\")"
        n137 = Unbundle By Name(w266) -> ("Core.Current VI Reference"=w265:refnum<vi>)
        n138 = case shown="\"Minimize\", \"Minimized\"" w264 {
          tunnel: w268 -> [w276 w291 w302 w315 w328]
          tunnel: [w278 w292 w304 w317 w330] -> w267
          tunnel: w265 -> [w277 w289 w303 w316 w329]
          frame "Open", "Standard", Default {
            w271 = T3."Standard" ("State")
            n139 = property class="VI"(reference=w277, error in=w276) -> (reference out=w274:refnum<vi>, error out=w275:errorcluster, "FP.State"=w273:T3)
            n140 = Not Equal?(x=w273, y=w271) -> (x != y?=w272:bool)
            n141 = case shown="True" w272 {
              tunnel: [w282 w284] -> w278
              tunnel: w275 -> [w281 w284]
              tunnel: w274 -> [w280 _]
              tunnel: w271 -> [w279 _]
              frame True {
                n142 = invoke class="VI" method="FP.Open"(reference=w280, error in=w281, "Activate"=TRUE, "State"=w279) -> (error out=w282:errorcluster)  [unwired: 1 in, 4 out]
              }
              frame False {
              }
            }
          }
          frame "Close", "Closed" {
            n143 = property class="VI"(reference=w289, error in=w291) -> (reference out=w288:refnum<vi>, error out=w290:errorcluster, "FP.State"=w286:T3)
            n144 = Not Equal?(x=w286, y=T3."Closed" ("Front Panel Window:State")) -> (x != y?=w285:bool)
            n145 = case shown="True" w285 {
              tunnel: [w293 w296] -> w292
              tunnel: w290 -> [w293 w295]
              tunnel: w288 -> [_ w294]
              frame False {
              }
              frame True {
                n146 = invoke class="VI" method="FP.Close"(reference=w294, error in=w295) -> (error out=w296:errorcluster)  [unwired: 1 in, 2 out]
              }
            }
          }
          frame "Hidden", "Hide" {
            w297 = T3."Hidden" ("State")
            n147 = property class="VI"(reference=w303, error in=w302) -> (reference out=w300:refnum<vi>, error out=w301:errorcluster, "FP.State"=w299:T3)
            n148 = Not Equal?(x=w299, y=w297) -> (x != y?=w298:bool)
            n149 = case shown="True" w298 {
              tunnel: [w308 w309] -> w304
              tunnel: w301 -> [w307 w309]
              tunnel: w300 -> [w306 _]
              tunnel: w297 -> [w305 _]
              frame True {
                n150 = invoke class="VI" method="FP.Open"(reference=w306, error in=w307, "State"=w305) -> (error out=w308:errorcluster)  [unwired: 2 in, 4 out]
              }
              frame False {
              }
            }
          }
          frame "Minimize", "Minimized" {
            w310 = T3."Minimized" ("State")
            n151 = property class="VI"(reference=w316, error in=w315) -> (reference out=w313:refnum<vi>, error out=w314:errorcluster, "FP.State"=w312:T3)
            n152 = Not Equal?(x=w312, y=w310) -> (x != y?=w311:bool)
            n153 = case shown="True" w311 {
              tunnel: [w321 w322] -> w317
              tunnel: w314 -> [w320 w322]
              tunnel: w313 -> [w319 _]
              tunnel: w310 -> [w318 _]
              frame True {
                n154 = invoke class="VI" method="FP.Open"(reference=w319, error in=w320, "State"=w318) -> (error out=w321:errorcluster)  [unwired: 2 in, 4 out]
              }
              frame False {
              }
            }
          }
          frame "Maximize", "Maximized" {
            w323 = T3."Maximized" ("State")
            n155 = property class="VI"(reference=w329, error in=w328) -> (reference out=w326:refnum<vi>, error out=w327:errorcluster, "FP.State"=w325:T3)
            n156 = Not Equal?(x=w325, y=w323) -> (x != y?=w324:bool)
            n157 = case shown="True" w324 {
              tunnel: [w334 w335] -> w330
              tunnel: w327 -> [w333 w335]
              tunnel: w326 -> [w332 _]
              tunnel: w323 -> [w331 _]
              frame True {
                n158 = invoke class="VI" method="FP.Open"(reference=w332, error in=w333, "State"=w331) -> (error out=w334:errorcluster)  [unwired: 2 in, 4 out]
              }
              frame False {
              }
            }
          }
        }
        n159 = call <vilib>:"Add State(s) to Queue__JKI_lib_State_Machine.vi"("State(s) in (\"\")"=w270) -> ("States Out"=w269:string)  [unwired: 14 in]
      }
      frame "---------- Macro ----------" {
        # "Do not put any code in this frame.\n(It is a separator no-op. You can make a copy of this frame to create a new Macro frame)"
        n160 = call <vilib>:"Add State(s) to Queue__JKI_lib_State_Machine.vi"("State(s) in (\"\")"=w339) -> ("States Out"=w338:string)  [unwired: 14 in]
      }
      frame "Macro: Initialize" {
        w340 = "Data: Initialize\nInitialize Core Data\nUI: Initialize\nUI: Front Panel State >> Open\n\nCFSSL: Find EXE\nCFSSL: Load Certification Authority\nCFSSL: Read CA Certificates\nCFSSL: Validate CA Certificates\nCFSSL: Create Temp Folder\nUI: List Certificates\nUI: Display Selected Certificate\nUI: Refresh"  # Data: Initialize Initialize Core Data UI: Initialize UI: Front Panel State >> Open  CFSSL: Find EXE CFSSL: Load Certification Authority CFSSL: Read CA Certificates CFSSL: Validate CA Certificates CFSSL: Create Temp Folder UI: List Certificates UI: Display Selected Certificate UI: Refresh
        # "Initialization Macro\n(This is called once, when the VI starts)"
        n161 = call <vilib>:"Add State(s) to Queue__JKI_lib_State_Machine.vi"("State(s) in Front (\"\")"=w340, "State(s) in (\"\")"=w344) -> ("States Out"=w343:string)  [unwired: 13 in]
      }
      frame "Macro: Generate Certification Authority" {
        n162 = call <vilib>:"Add State(s) to Queue__JKI_lib_State_Machine.vi"("State(s) in Front (\"\")"="CFSSL: Create Temp Folder\nCFSSL: Prepare CA Request File\nCFSSL: Generate Certification Authority\nCFSSL: Save CA Certificate\nCFSSL: Load Certification Authority\nCFSSL: Read CA Certificates\nCFSSL: Validate CA Certificates\nUI: Refresh\nUI: List Certificates\nUI: Display Selected Certificate", "State(s) in (\"\")"=w349) -> ("States Out"=w348:string)  [unwired: 13 in]
      }
      frame "Macro: Generate Server Certificate" {
        n163 = Bundle By Name(cluster=w353, "Processing Queue"="Servers") -> (w352:T11)
        n164 = call <vilib>:"Add State(s) to Queue__JKI_lib_State_Machine.vi"("State(s) in Front (\"\")"="CFSSL: Create Temp Folder\nCFSSL: Prepare Gencert Config File\nCFSSL: Copy Temporary CA Certificate\n\nMacro: Process Next Server", "State(s) in (\"\")"=w357, "State(s) at Back (\"\")"="UI: Refresh\nUI: List Certificates\nUI: Display Selected Certificate") -> ("States Out"=w356:string)  [unwired: 12 in]
      }
      frame "Macro: Export Root Bundle" {
        n165 = call <vilib>:"Add State(s) to Queue__JKI_lib_State_Machine.vi"("State(s) in Front (\"\")"="CFSSL: Export Root Certificate\nCFSSL: Export Root Private Key\nCFSSL: Export Root Signing Request", "State(s) in (\"\")"=w362) -> ("States Out"=w361:string)  [unwired: 13 in]
      }
      frame "Macro: Process Next Server" {
        n166 = Unbundle By Name(w368) -> ("Processing Queue"=w367:cluster{"hosts":string[], "name":string}[])
        n167 = Empty Array?(array=w367) -> (empty?=w366:bool)
        n168 = Select(t="UI: Refresh", s=w366, f="CFSSL: Load Next Server\nCFSSL: Prepare Server Request File\nCFSSL: Generate Server Certificate\nCFSSL: Save Temporary Server Certificate\nMacro: Process Next Server") -> (s? t:f=w363:string)
        n169 = call <vilib>:"Add State(s) to Queue__JKI_lib_State_Machine.vi"("State(s) in Front (\"\")"=w363, "State(s) in (\"\")"=w371) -> ("States Out"=w370:string)  [unwired: 13 in]
      }
      frame "Macro: Export Server Bundle" {
        n170 = call <vilib>:"Add State(s) to Queue__JKI_lib_State_Machine.vi"("State(s) in Front (\"\")"="CFSSL: Export Server Certificate\nCFSSL: Export Server Private Key\nCFSSL: Export Server Signing Request", "State(s) in (\"\")"=w376) -> ("States Out"=w375:string)  [unwired: 13 in]
      }
      frame "Macro: Exit" {
        # "Exit Macro\n(This is called once, when the VI exits)"
        n171 = Unbundle By Name(w384) -> ("Core.Close Panel on Exit?"=w383:bool)
        n172 = Select(t="UI: Front Panel State >> Close", s=w383, f="") -> (s? t:f=w380:string)
        n173 = call <vilib>:"Add State(s) to Queue__JKI_lib_State_Machine.vi"("State(s) in Front (\"\")"="CFSSL: Delete Temp Folder", "State(s) in (\"\")"=w380, "State(s) at Back (\"\")"="Data: Cleanup\nExit") -> ("States Out"=w378:string)  [unwired: 12 in]
        n174 = call <vilib>:"Add State(s) to Queue__JKI_lib_State_Machine.vi"("State(s) in Front (\"\")"=w378, "State(s) in (\"\")"=w387) -> ("States Out"=w386:string)  [unwired: 13 in]
      }
      frame "---------- Cloudflare SSL ----------" {
        n175 = call <vilib>:"Add State(s) to Queue__JKI_lib_State_Machine.vi"("State(s) in (\"\")"=w391) -> ("States Out"=w390:string)  [unwired: 14 in]
      }
      frame "CFSSL: Find EXE" {
        n176 = call "LVOS Certificates Folder.vi"() -> ("cfssl path"=w393:path)  [unwired: 10 in, 1 out]
        n177 = call <userlib>:"Create Dir if Non-Existant__ogtk.vi"("Directory Path"=w393) -> ("dup Directory Path"=w394:path)  [unwired: 8 in, 2 out]
        n178 = Build Path(base path=w394, name or relative path=path "cfssl.exe") -> (appended path=w396:path)
        n179 = call-poly <userlib>:"File Exists__ogtk.vi"("file path"=w396) -> ("is directory"=w400:bool, "exists"=w399:bool)  [unwired: 6 in]
        n180 = Compound Arithmetic op=OR(invert w400, w399) -> (w398:bool)
        n181 = Select(t=w396, s=w398, f=path "") -> (s? t:f=w397:path)
        n182 = Bundle By Name(cluster=w402, "cfssl path"=w397) -> (w401:T11)
        n183 = call <vilib>:"Add State(s) to Queue__JKI_lib_State_Machine.vi"("State(s) in (\"\")"=w405) -> ("States Out"=w404:string)  [unwired: 14 in]
      }
      frame "CFSSL: Create Temp Folder" {
        n184 = call <userlib>:"Temporary Directory__ogtk.vi"("Relative path (.)"=path "LV_CFSSL") -> ("Temporary Directory (+ Relative)"=w409:path)
        n185 = call <userlib>:"Create Dir if Non-Existant__ogtk.vi"("error in (no error)"=w408, "Directory Path"=w409) -> ("error out"=w407:errorcluster, "dup Directory Path"=w406:path)  [unwired: 7 in, 1 out]
        n186 = Bundle By Name(cluster=w412, "temp folder"=w406) -> (w411:T11)
        n187 = call <vilib>:"Add State(s) to Queue__JKI_lib_State_Machine.vi"("State(s) in (\"\")"=w414) -> ("States Out"=w413:string)  [unwired: 14 in]
      }
      frame "CFSSL: Delete Temp Folder" {
        n188 = Unbundle By Name(w422) -> ("temp folder"=w416:path)
        n189 = Empty String/Path?(string/path=w416) -> (empty?=w415:bool)
        n190 = call-poly <userlib>:"File Exists__ogtk.vi"("file path"=w416) -> ("is directory"=w420:bool, "exists"=w421:bool)  [unwired: 6 in]
        n191 = Compound Arithmetic op=AND(w420, w421, invert w415) -> (w419:bool)
        n192 = case shown="True" w419 {
          tunnel: w416 -> [_ w429]
          tunnel: [w425 w427] -> w418
          tunnel: w417 -> [w425 w428]
          frame False {
          }
          frame True {
            w426 = TRUE ("Recursive? (FALSE)")
            n193 = call <userlib>:"Delete Recursive__ogtk.vi"("error in (no error)"=w428, "Ignore Read-Only? (FALSE)"=w426, "Recursive? (FALSE)"=w426, "Path"=w429) -> ("error out"=w427:errorcluster)  [unwired: 6 in, 1 out]
          }
        }
        n194 = call <vilib>:"Add State(s) to Queue__JKI_lib_State_Machine.vi"("State(s) in (\"\")"=w424) -> ("States Out"=w423:string)  [unwired: 14 in]
      }
      frame "CFSSL: Load Certification Authority" {
        n195 = Unbundle By Name(w447) -> ("Certificates Folder"=w431:path)
        n196 = Build Path(base path=w431, name or relative path="root.crt") -> (appended path=w432:path)
        n197 = Build Path(base path=w431, name or relative path="root-key.pem") -> (appended path=w430:path)
        n198 = call-poly <userlib>:"File Exists__ogtk.vi"("file path"=w432) -> ("is directory"=w445:bool, "exists"=w444:bool)  [unwired: 6 in]
        n199 = Empty String/Path?(string/path=w432) -> (empty?=w443:bool)
        n200 = call-poly <userlib>:"File Exists__ogtk.vi"("file path"=w430) -> ("is directory"=w435:bool, "exists"=w436:bool)  [unwired: 6 in]
        n201 = Empty String/Path?(string/path=w430) -> (empty?=w437:bool)
        n202 = Compound Arithmetic op=AND(invert w445, w444, invert w443) -> (w442:bool)
        n203 = Compound Arithmetic op=AND(invert w435, w436, invert w437) -> (w438:bool)
        n204 = Select(t=w432, s=w442, f=path "") -> (s? t:f=w440:path)
        n205 = Select(t=w430, s=w438, f=path "") -> (s? t:f=w433:path)
        n206 = Bundle By Name(cluster=w447, "Root Certificate"=w440, "Root Private Key"=w433) -> (w448:T11)
        n207 = call <vilib>:"Add State(s) to Queue__JKI_lib_State_Machine.vi"("State(s) in (\"\")"=w451) -> ("States Out"=w450:string)  [unwired: 14 in]
      }
      frame "CFSSL: Generate Certification Authority" {
        n208 = Unbundle By Name(w455) -> ("cfssl path"=w461:path, "temp folder"=w460:path)
        n209 = Format Into String(format string="\"%s\" gencert -initca csr-ca.json", w461) -> (resulting string=w463:string)  [unwired: 2 in, 1 out]
        n210 = call <vilib>:"System Exec.vi"("run minimized? (F)"=TRUE, "error in (no error)"=w453, "working directory"=w460, "command line"=w463) -> ("error out"=w458:errorcluster, "standard output"=w459:string)  [unwired: 4 in, 2 out]
        n211 = Unbundle By Name(w455) -> ("CA"=w454:T10)
        n212 = Unflatten From JSON(JSON string=w459, type and defaults=w454, error in (no error)=w458) -> (value=w457:T10, error out=w452:errorcluster)  [unwired: 4 in]
        n213 = Bundle By Name(cluster=w455, "CA"=w457) -> (w456:T11)
        n214 = call <vilib>:"Add State(s) to Queue__JKI_lib_State_Machine.vi"("State(s) in (\"\")"=w466) -> ("States Out"=w465:string)  [unwired: 14 in]
      }
      frame "CFSSL: Generate Server Certificate" {
        n215 = Unbundle By Name(w471) -> ("cfssl path"=w477:path, "temp folder"=w476:path)
        n216 = Format Into String(format string="\"%s\" gencert -ca ca.pem -ca-key ca-key.pem -config config.json csr-server.json" ("command line"), w477) -> (resulting string=w478:string)  [unwired: 2 in, 1 out]
        n217 = call <vilib>:"System Exec.vi"("run minimized? (F)"=TRUE, "error in (no error)"=w469, "working directory"=w476, "command line"=w478) -> ("error out"=w474:errorcluster, "standard output"=w475:string)  [unwired: 4 in, 2 out]
        n218 = Unbundle By Name(w471) -> ("Server"=w470:T10)
        n219 = Unflatten From JSON(JSON string=w475, type and defaults=w470, error in (no error)=w474) -> (value=w473:T10, error out=w468:errorcluster)  [unwired: 4 in]
        n220 = Bundle By Name(cluster=w471, "Server"=w473) -> (w472:T11)
        n221 = call <vilib>:"Add State(s) to Queue__JKI_lib_State_Machine.vi"("State(s) in (\"\")"=w481) -> ("States Out"=w480:string)  [unwired: 14 in]
      }
      frame "CFSSL: Prepare CA Request File" {
        (unwired) "{\n    \"CN\": \"lvtls-ca.example\",\n    \"hosts\": [\"lvtls-ca.example\"],\n    \"key\": {\"algo\": \"ecdsa\", \"size\": 256},\n    \"names\": [],\n    \"ca\": {\"pathlen\": 1, \"expiry\": \"143800h\"}\n}" ("name or relative path")
        # "https://github.com/cloudflare/cfssl/wiki/Creating-a-new-CSR"
        n222 = Unbundle By Name(w502) -> ("temp folder"=w501:path)
        n223 = call-poly <userlib>:"Build Path__ogtk.vi"("name or relative path"="csr-ca.json", "base path"=w501) -> ("appended path"=w490:path)
        n224 = Bundle By Name(cluster=T6 {"CN"="", "hosts"=[], "key"={"algo"="ecdsa", "size"=256}, "ca"={"pathlen"=0, "expiry"=""}} ("CSR"), "CN"="Common Name", "hosts"="Hosts", "key.algo"="ecdsa", "key.size"=u32 256, "ca.pathlen"=u8 1, "ca.expiry"="143800h") -> (w496:T6)
        n225 = Flatten To JSON(anything=w496, error in (no error)=w483) -> (JSON string=w488:string, 11:w484:errorcluster)  [unwired: 1 in]
        n226 = Open/Create/Replace File(file path (use dialog)=w490, error in=w484, operation (0:open)=T5."replace or create") -> (refnum out=w489:refnum<file>, error out=w491:errorcluster)  [unwired: 3 in, 1 out]
        n227 = Write to Text File(file (use dialog)=w489, text=w488, error in=w491) -> (refnum out=w485:refnum<file>, error out=w486:errorcluster)  [unwired: 1 in, 1 out]
        n228 = Close File(refnum=w485, error in=w486) -> (error out=w482:errorcluster)  [unwired: 1 out]
        n229 = call <vilib>:"Add State(s) to Queue__JKI_lib_State_Machine.vi"("State(s) in (\"\")"=w504) -> ("States Out"=w503:string)  [unwired: 14 in]
      }
      frame "CFSSL: Prepare Server Request File" {
        (unwired) "{\n    \"CN\": \"lvtls.example\",\n    \"hosts\": [\"lvtls.example\"],\n    \"key\": {\"algo\": \"ecdsa\", \"size\": 256},\n    \"names\": []\n}" ("name or relative path")
        # "https://github.com/cloudflare/cfssl/wiki/Creating-a-new-CSR"
        n230 = Unbundle By Name(w523) -> ("temp folder"=w522:path, "Active CN"=w506:string, "Active Hosts"=w505:string[])
        n231 = call-poly <userlib>:"Build Path__ogtk.vi"("name or relative path"="csr-server.json", "base path"=w522) -> ("appended path"=w519:path)
        n232 = Bundle By Name(cluster=T9 {"CN"="", "hosts"=[], "key"={"algo"="ecdsa", "size"=256}} ("CSR"), "CN"=w506, "hosts"=w505, "key.algo"="ecdsa", "key.size"=u32 256) -> (w508:T9)
        n233 = Flatten To JSON(anything=w508, error in (no error)=w512) -> (JSON string=w517:string, 11:w513:errorcluster)  [unwired: 1 in]
        n234 = Open/Create/Replace File(file path (use dialog)=w519, error in=w513, operation (0:open)=T5."replace or create") -> (refnum out=w518:refnum<file>, error out=w520:errorcluster)  [unwired: 3 in, 1 out]
        n235 = Write to Text File(file (use dialog)=w518, text=w517, error in=w520) -> (refnum out=w514:refnum<file>, error out=w515:errorcluster)  [unwired: 1 in, 1 out]
        n236 = Close File(refnum=w514, error in=w515) -> (error out=w511:errorcluster)  [unwired: 1 out]
        n237 = call <vilib>:"Add State(s) to Queue__JKI_lib_State_Machine.vi"("State(s) in (\"\")"=w525) -> ("States Out"=w524:string)  [unwired: 14 in]
      }
      frame "CFSSL: Copy Temporary CA Certificate" {
        n238 = Unbundle By Name(w535) -> ("Root Certificate"=w539:path, "temp folder"=w540:path)
        n239 = Unbundle By Name(w535) -> ("Root Private Key"=w532:path, "temp folder"=w530:path)
        n240 = call-poly <userlib>:"Build Path__ogtk.vi"("name or relative path"="ca-key.pem", "base path"=w530) -> ("appended path"=w533:path)
        n241 = call-poly <userlib>:"Build Path__ogtk.vi"("name or relative path"="ca.pem", "base path"=w540) -> ("appended path"=w537:path)
        n242 = call <userlib>:"Copy with Options__ogtk.vi"("error in (no error)"=w529, "Replace Mode (Never)"=enum16{"Never", "Always", "If Newer"}."Always", "target path"=w533, "source path"=w532) -> ("error out"=w526:errorcluster)  [unwired: 6 in, 1 out]
        n243 = call <userlib>:"Copy with Options__ogtk.vi"("error in (no error)"=w529, "Replace Mode (Never)"=enum16{"Never", "Always", "If Newer"}."Always", "target path"=w537, "source path"=w539) -> ("error out"=w527:errorcluster)  [unwired: 6 in, 1 out]
        n244 = Merge Errors(w527, w526) -> (w528:errorcluster)
        n245 = call <vilib>:"Add State(s) to Queue__JKI_lib_State_Machine.vi"("State(s) in (\"\")"=w542) -> ("States Out"=w541:string)  [unwired: 14 in]
      }
      frame "CFSSL: Load Next Server" {
        n246 = Unbundle By Name(w547) -> ("Processing Queue"=w546:cluster{"hosts":string[], "name":string}[])
        n247 = Delete From Array(array=w546) -> (deleted portion=w544:cluster{"hosts":string[], "name":string}, array with subset deleted=w545:cluster{"hosts":string[], "name":string}[])  [unwired: 2 in]
        n248 = Unbundle By Name(w544) -> ("name"=w549:string, "hosts"=w548:string[])
        n249 = Bundle By Name(cluster=w547, "Processing Queue"=w545, "Active CN"=w549, "Active Hosts"=w548) -> (w550:T11)
        n250 = call <vilib>:"Add State(s) to Queue__JKI_lib_State_Machine.vi"("State(s) in (\"\")"=w552) -> ("States Out"=w551:string)  [unwired: 14 in]
      }
      frame "CFSSL: Prepare Gencert Config File" {
        n251 = Unbundle By Name(w564) -> ("temp folder"=w563:path)
        n252 = call-poly <userlib>:"Build Path__ogtk.vi"("name or relative path"="config.json", "base path"=w563) -> ("appended path"=w560:path)
        n253 = Open/Create/Replace File(file path (use dialog)=w560, error in=w553, operation (0:open)=T5."replace or create") -> (refnum out=w559:refnum<file>, error out=w561:errorcluster)  [unwired: 3 in, 1 out]
        n254 = Write to Text File(file (use dialog)=w559, text="{\n  \"signing\": {\n       \"default\": {\n           \"expiry\": \"143800h\", \n           \"usages\": [\"server auth\"]\n        }\n    }\n}" ("name or relative path"), error in=w561) -> (refnum out=w556:refnum<file>, error out=w557:errorcluster)  [unwired: 1 in, 1 out]
        n255 = Close File(refnum=w556, error in=w557) -> (error out=w555:errorcluster)  [unwired: 1 out]
        n256 = call <vilib>:"Add State(s) to Queue__JKI_lib_State_Machine.vi"("State(s) in (\"\")"=w566) -> ("States Out"=w565:string)  [unwired: 14 in]
      }
      frame "CFSSL: Save CA Certificate" {
        w575 = T5."replace or create with confirmation" ("operation (0:open)")
        n257 = Unbundle By Name(w567) -> ("Certificates Folder"=w588:path)
        n258 = Unbundle By Name(w567) -> ("CA.cert"=w587:string)
        n259 = Unbundle By Name(w567) -> ("CA.key"=w576:string)
        n260 = Unbundle By Name(w567) -> ("CA.csr"=w577:string)
        n261 = call-poly <userlib>:"Build Path__ogtk.vi"("name or relative path"="root.csr", "base path"=w588) -> ("appended path"=w582:path)
        n262 = call-poly <userlib>:"Build Path__ogtk.vi"("name or relative path"="root.crt", "base path"=w588) -> ("appended path"=w569:path)
        n263 = call-poly <userlib>:"Build Path__ogtk.vi"("name or relative path"="root-key.pem", "base path"=w588) -> ("appended path"=w568:path)
        n264 = Open/Create/Replace File(file path (use dialog)=w582, operation (0:open)=w575) -> (refnum out=w584:refnum<file>, error out=w583:errorcluster)  [unwired: 4 in, 1 out]
        n265 = Open/Create/Replace File(file path (use dialog)=w568, operation (0:open)=w575) -> (refnum out=w580:refnum<file>, error out=w581:errorcluster)  [unwired: 4 in, 1 out]
        n266 = Open/Create/Replace File(file path (use dialog)=w569, operation (0:open)=w575) -> (refnum out=w593:refnum<file>, error out=w594:errorcluster)  [unwired: 4 in, 1 out]
        n267 = Write to Text File(file (use dialog)=w584, text=w577, error in=w583) -> (refnum out=w586:refnum<file>, error out=w585:errorcluster)  [unwired: 1 in, 1 out]
        n268 = Write to Text File(file (use dialog)=w580, text=w576, error in=w581) -> (refnum out=w578:refnum<file>, error out=w579:errorcluster)  [unwired: 1 in, 1 out]
        n269 = Write to Text File(file (use dialog)=w593, text=w587, error in=w594) -> (refnum out=w591:refnum<file>, error out=w592:errorcluster)  [unwired: 1 in, 1 out]
        n270 = Close File(refnum=w586, error in=w585) -> (error out=w572:errorcluster)  [unwired: 1 out]
        n271 = Close File(refnum=w578, error in=w579) -> (error out=w571:errorcluster)  [unwired: 1 out]
        n272 = Close File(refnum=w591, error in=w592) -> (error out=w573:errorcluster)  [unwired: 1 out]
        n273 = Merge Errors(w574, w573, w572, w571) -> (w570:errorcluster)
        n274 = call <vilib>:"Add State(s) to Queue__JKI_lib_State_Machine.vi"("State(s) in (\"\")"=w597) -> ("States Out"=w596:string)  [unwired: 14 in]
      }
      frame "CFSSL: Read CA Certificates" {
        n275 = Unbundle By Name(w613) -> ("Certificates Folder"=w614:path)
        n276 = call-poly <userlib>:"Build Path__ogtk.vi"("name or relative path"="root-key.pem", "base path"=w614) -> ("appended path"=w599:path)
        n277 = call-poly <userlib>:"Build Path__ogtk.vi"("name or relative path"="root.crt", "base path"=w614) -> ("appended path"=w604:path)
        n278 = call-poly <userlib>:"File Exists__ogtk.vi"("file path"=w604) -> ("is directory"=w607:bool, "exists"=w606:bool)  [unwired: 6 in]
        n279 = Empty String/Path?(string/path=w604) -> (empty?=w605:bool)
        n280 = call-poly <userlib>:"File Exists__ogtk.vi"("file path"=w599) -> ("is directory"=w600:bool, "exists"=w601:bool)  [unwired: 6 in]
        n281 = Empty String/Path?(string/path=w599) -> (empty?=w602:bool)
        n282 = Compound Arithmetic op=AND(invert w607, w606, invert w605) -> (w603:bool)
        n283 = Compound Arithmetic op=AND(invert w600, w601, invert w602) -> (w598:bool)
        n284 = case shown="True" w603 {
          tunnel: w604 -> [_ w637]
          tunnel: [_ w633] -> w611
          tunnel: [_ w630] -> w610
          frame False {
          }
          frame True {
            n285 = Open/Create/Replace File(file path (use dialog)=w637, operation (0:open)=T5."open", access (0:read/write)=enum16{"read/write", "read-only", "write-only"}."read-only") -> (refnum out=w636:refnum<file>, error out=w638:errorcluster)  [unwired: 3 in, 1 out]
            n286 = Read from Text File(file (use dialog)=w636, error in=w638) -> (refnum out=w634:refnum<file>, text=w633:string, error out=w635:errorcluster)  [unwired: 2 in, 1 out]
            n287 = Close File(refnum=w634, error in=w635) -> (error out=w630:errorcluster)  [unwired: 1 out]
          }
        }
        n288 = case shown="True" w598 {
          tunnel: w599 -> [_ w625]
          tunnel: [_ w624] -> w609
          tunnel: [_ w621] -> w608
          frame False {
          }
          frame True {
            n289 = Open/Create/Replace File(file path (use dialog)=w625, operation (0:open)=T5."open", access (0:read/write)=enum16{"read/write", "read-only", "write-only"}."read-only") -> (refnum out=w627:refnum<file>, error out=w626:errorcluster)  [unwired: 3 in, 1 out]
            n290 = Read from Text File(file (use dialog)=w627, error in=w626) -> (refnum out=w629:refnum<file>, text=w621:string, error out=w628:errorcluster)  [unwired: 2 in, 1 out]
            n291 = Close File(refnum=w629, error in=w628) -> (error out=w624:errorcluster)  [unwired: 1 out]
          }
        }
        n292 = Bundle By Name(cluster=w613, "CA.cert"=w611, "CA.key"=w608) -> (w612:T11)
        n293 = Merge Errors(w616, w610, w609) -> (w615:errorcluster)
        n294 = call <vilib>:"Add State(s) to Queue__JKI_lib_State_Machine.vi"("State(s) in (\"\")"=w620) -> ("States Out"=w619:string)  [unwired: 14 in]
      }
      frame "CFSSL: Validate CA Certificates" {
        n295 = Unbundle By Name(w642) -> ("Root Certificate"=w640:path, "Root Private Key"=w639:path)  [unwired: 2 out]
        n296 = Bundle By Name(cluster=w642, "Root Certificate"=w640, "Root Private Key"=w639) -> (w641:T11)
        n297 = Merge Errors(w644) -> (w643:errorcluster)
        n298 = call <vilib>:"Add State(s) to Queue__JKI_lib_State_Machine.vi"("State(s) in (\"\")"=w646) -> ("States Out"=w645:string)  [unwired: 14 in]
      }
      frame "CFSSL: Save Temporary CA Certificate" {
        w647 = T5."replace or create" ("operation (0:open)")
        n299 = Unbundle By Name(w659) -> ("temp folder"=w660:path)
        n300 = Unbundle By Name(w659) -> ("CA.cert"=w658:string)
        n301 = Unbundle By Name(w659) -> ("CA.key"=w652:string)
        n302 = call-poly <userlib>:"Build Path__ogtk.vi"("name or relative path"="root.crt", "base path"=w660) -> ("appended path"=w665:path)
        n303 = call-poly <userlib>:"Build Path__ogtk.vi"("name or relative path"="root-key.pem", "base path"=w660) -> ("appended path"=w653:path)
        n304 = Open/Create/Replace File(file path (use dialog)=w653, operation (0:open)=w647) -> (refnum out=w656:refnum<file>, error out=w657:errorcluster)  [unwired: 4 in, 1 out]
        n305 = Open/Create/Replace File(file path (use dialog)=w665, operation (0:open)=w647) -> (refnum out=w664:refnum<file>, error out=w666:errorcluster)  [unwired: 4 in, 1 out]
        n306 = Write to Text File(file (use dialog)=w656, text=w652, error in=w657) -> (refnum out=w654:refnum<file>, error out=w655:errorcluster)  [unwired: 1 in, 1 out]
        n307 = Write to Text File(file (use dialog)=w664, text=w658, error in=w666) -> (refnum out=w662:refnum<file>, error out=w663:errorcluster)  [unwired: 1 in, 1 out]
        n308 = Close File(refnum=w654, error in=w655) -> (error out=w649:errorcluster)  [unwired: 1 out]
        n309 = Close File(refnum=w662, error in=w663) -> (error out=w650:errorcluster)  [unwired: 1 out]
        n310 = Merge Errors(w651, w650, w649) -> (w648:errorcluster)
        n311 = call <vilib>:"Add State(s) to Queue__JKI_lib_State_Machine.vi"("State(s) in (\"\")"=w669) -> ("States Out"=w668:string)  [unwired: 14 in]
      }
      frame "CFSSL: Save Temporary Server Certificate" {
        w689 = T5."replace or create" ("operation (0:open)")
        n312 = Unbundle By Name(w684) -> ("Certificates Folder"=w680:path, "Active CN"=w676:string)
        n313 = Unbundle By Name(w684) -> ("Certificates Folder"=w679:path, "Active CN"=w683:string, "Server.key"=w678:string)
        n314 = Unbundle By Name(w684) -> ("Server.cert"=w670:string, "CA.cert"=w672:string)
        n315 = Format Into String(format string="%s-key.pem", w683) -> (resulting string=w681:string)  [unwired: 2 in, 1 out]
        n316 = Format Into String(format string="%s.crt", w676) -> (resulting string=w677:string)  [unwired: 2 in, 1 out]
        n317 = call-poly <userlib>:"Build Path__ogtk.vi"("name or relative path"=w677, "base path"=w680) -> ("appended path"=w698:path)
        n318 = call-poly <userlib>:"Build Path__ogtk.vi"("name or relative path"=w681, "base path"=w679) -> ("appended path"=w690:path)
        n319 = Open/Create/Replace File(file path (use dialog)=w690, operation (0:open)=w689) -> (refnum out=w693:refnum<file>, error out=w694:errorcluster)  [unwired: 4 in, 1 out]
        n320 = Open/Create/Replace File(file path (use dialog)=w698, operation (0:open)=w689) -> (refnum out=w697:refnum<file>, error out=w699:errorcluster)  [unwired: 4 in, 1 out]
        n321 = Write to Text File(file (use dialog)=w693, text=w678, error in=w694) -> (refnum out=w691:refnum<file>, error out=w692:errorcluster)  [unwired: 1 in, 1 out]
        n322 = Format Into String(format string="%s%s%s", w670, "\n", w672) -> (resulting string=w671:string)  [unwired: 2 in, 1 out]
        n323 = Close File(refnum=w691, error in=w692) -> (error out=w686:errorcluster)  [unwired: 1 out]
        n324 = Write to Text File(file (use dialog)=w697, text=w671, error in=w699) -> (refnum out=w695:refnum<file>, error out=w696:errorcluster)  [unwired: 1 in, 1 out]
        n325 = Close File(refnum=w695, error in=w696) -> (error out=w687:errorcluster)  [unwired: 1 out]
        n326 = Merge Errors(w688, w687, w686) -> (w685:errorcluster)
        n327 = call <vilib>:"Add State(s) to Queue__JKI_lib_State_Machine.vi"("State(s) in (\"\")"=w701) -> ("States Out"=w700:string)  [unwired: 14 in]
      }
      frame "CFSSL: Export Root Private Key" {
        n328 = Unbundle By Name(w710) -> ("Certificates Folder"=w711:path, "Root name"=w704:string)
        n329 = Unbundle By Name(w710) -> ("CA.key"=w709:string)
        n330 = call-poly <userlib>:"Convert File Extension__ogtk.vi"("new ending (none)"="pem" ("format string"), "file name"=w704) -> ("new filename"=w702:string)  [unwired: 1 out]
        n331 = call-poly <userlib>:"Build Path__ogtk.vi"("name or relative path"=w702, "base path"=w711) -> ("appended path"=w715:path)
        n332 = Open/Create/Replace File(file path (use dialog)=w715, operation (0:open)=T5."replace or create with confirmation") -> (refnum out=w714:refnum<file>, error out=w716:errorcluster)  [unwired: 4 in, 1 out]
        n333 = Write to Text File(file (use dialog)=w714, text=w709, error in=w716) -> (refnum out=w712:refnum<file>, error out=w713:errorcluster)  [unwired: 1 in, 1 out]
        n334 = Close File(refnum=w712, error in=w713) -> (error out=w706:errorcluster)  [unwired: 1 out]
        n335 = Merge Errors(w707, w706) -> (w705:errorcluster)
        n336 = call <vilib>:"Add State(s) to Queue__JKI_lib_State_Machine.vi"("State(s) in (\"\")"=w718) -> ("States Out"=w717:string)  [unwired: 14 in]
      }
      frame "CFSSL: Export Root Certificate" {
        n337 = Unbundle By Name(w727) -> ("Certificates Folder"=w728:path, "Root name"=w721:string)
        n338 = Unbundle By Name(w727) -> ("CA.cert"=w726:string)
        n339 = call-poly <userlib>:"Convert File Extension__ogtk.vi"("new ending (none)"="crt" ("format string"), "file name"=w721) -> ("new filename"=w719:string)  [unwired: 1 out]
        n340 = call-poly <userlib>:"Build Path__ogtk.vi"("name or relative path"=w719, "base path"=w728) -> ("appended path"=w732:path)
        n341 = Open/Create/Replace File(file path (use dialog)=w732, operation (0:open)=T5."replace or create with confirmation") -> (refnum out=w731:refnum<file>, error out=w733:errorcluster)  [unwired: 4 in, 1 out]
        n342 = Write to Text File(file (use dialog)=w731, text=w726, error in=w733) -> (refnum out=w729:refnum<file>, error out=w730:errorcluster)  [unwired: 1 in, 1 out]
        n343 = Close File(refnum=w729, error in=w730) -> (error out=w723:errorcluster)  [unwired: 1 out]
        n344 = Merge Errors(w724, w723) -> (w722:errorcluster)
        n345 = call <vilib>:"Add State(s) to Queue__JKI_lib_State_Machine.vi"("State(s) in (\"\")"=w735) -> ("States Out"=w734:string)  [unwired: 14 in]
      }
      frame "CFSSL: Export Root Signing Request" {
        n346 = Unbundle By Name(w744) -> ("Certificates Folder"=w745:path, "Root name"=w738:string)
        n347 = Unbundle By Name(w744) -> ("CA.csr"=w743:string)
        n348 = call-poly <userlib>:"Convert File Extension__ogtk.vi"("new ending (none)"="csr" ("format string"), "file name"=w738) -> ("new filename"=w736:string)  [unwired: 1 out]
        n349 = call-poly <userlib>:"Build Path__ogtk.vi"("name or relative path"=w736, "base path"=w745) -> ("appended path"=w749:path)
        n350 = Open/Create/Replace File(file path (use dialog)=w749, operation (0:open)=T5."replace or create with confirmation") -> (refnum out=w748:refnum<file>, error out=w750:errorcluster)  [unwired: 4 in, 1 out]
        n351 = Write to Text File(file (use dialog)=w748, text=w743, error in=w750) -> (refnum out=w746:refnum<file>, error out=w747:errorcluster)  [unwired: 1 in, 1 out]
        n352 = Close File(refnum=w746, error in=w747) -> (error out=w740:errorcluster)  [unwired: 1 out]
        n353 = Merge Errors(w741, w740) -> (w739:errorcluster)
        n354 = call <vilib>:"Add State(s) to Queue__JKI_lib_State_Machine.vi"("State(s) in (\"\")"=w752) -> ("States Out"=w751:string)  [unwired: 14 in]
      }
      frame "CFSSL: Export Server Certificate" {
        n355 = Unbundle By Name(w761) -> ("Certificates Folder"=w762:path, "Root name"=w755:string)
        n356 = Unbundle By Name(w761) -> ("Server.cert"=w760:string)
        n357 = call-poly <userlib>:"Convert File Extension__ogtk.vi"("new ending (none)"="cer" ("format string"), "file name"=w755) -> ("new filename"=w753:string)  [unwired: 1 out]
        n358 = call-poly <userlib>:"Build Path__ogtk.vi"("name or relative path"=w753, "base path"=w762) -> ("appended path"=w766:path)
        n359 = Open/Create/Replace File(file path (use dialog)=w766, operation (0:open)=T5."replace or create with confirmation") -> (refnum out=w765:refnum<file>, error out=w767:errorcluster)  [unwired: 4 in, 1 out]
        n360 = Write to Text File(file (use dialog)=w765, text=w760, error in=w767) -> (refnum out=w763:refnum<file>, error out=w764:errorcluster)  [unwired: 1 in, 1 out]
        n361 = Close File(refnum=w763, error in=w764) -> (error out=w757:errorcluster)  [unwired: 1 out]
        n362 = Merge Errors(w758, w757) -> (w756:errorcluster)
        n363 = call <vilib>:"Add State(s) to Queue__JKI_lib_State_Machine.vi"("State(s) in (\"\")"=w769) -> ("States Out"=w768:string)  [unwired: 14 in]
      }
      frame "CFSSL: Export Server Private Key" {
        n364 = Unbundle By Name(w778) -> ("Certificates Folder"=w779:path, "Root name"=w772:string)
        n365 = Unbundle By Name(w778) -> ("Server.key"=w777:string)
        n366 = call-poly <userlib>:"Convert File Extension__ogtk.vi"("new ending (none)"="pem" ("format string"), "file name"=w772) -> ("new filename"=w770:string)  [unwired: 1 out]
        n367 = call-poly <userlib>:"Build Path__ogtk.vi"("name or relative path"=w770, "base path"=w779) -> ("appended path"=w783:path)
        n368 = Open/Create/Replace File(file path (use dialog)=w783, operation (0:open)=T5."replace or create with confirmation") -> (refnum out=w782:refnum<file>, error out=w784:errorcluster)  [unwired: 4 in, 1 out]
        n369 = Write to Text File(file (use dialog)=w782, text=w777, error in=w784) -> (refnum out=w780:refnum<file>, error out=w781:errorcluster)  [unwired: 1 in, 1 out]
        n370 = Close File(refnum=w780, error in=w781) -> (error out=w774:errorcluster)  [unwired: 1 out]
        n371 = Merge Errors(w775, w774) -> (w773:errorcluster)
        n372 = call <vilib>:"Add State(s) to Queue__JKI_lib_State_Machine.vi"("State(s) in (\"\")"=w786) -> ("States Out"=w785:string)  [unwired: 14 in]
      }
      frame "CFSSL: Export Server Signing Request" {
        n373 = Unbundle By Name(w795) -> ("Certificates Folder"=w796:path, "Root name"=w789:string)
        n374 = Unbundle By Name(w795) -> ("Server.csr"=w794:string)
        n375 = call-poly <userlib>:"Convert File Extension__ogtk.vi"("new ending (none)"="csr" ("format string"), "file name"=w789) -> ("new filename"=w787:string)  [unwired: 1 out]
        n376 = call-poly <userlib>:"Build Path__ogtk.vi"("name or relative path"=w787, "base path"=w796) -> ("appended path"=w800:path)
        n377 = Open/Create/Replace File(file path (use dialog)=w800, operation (0:open)=T5."replace or create with confirmation") -> (refnum out=w799:refnum<file>, error out=w801:errorcluster)  [unwired: 4 in, 1 out]
        n378 = Write to Text File(file (use dialog)=w799, text=w794, error in=w801) -> (refnum out=w797:refnum<file>, error out=w798:errorcluster)  [unwired: 1 in, 1 out]
        n379 = Close File(refnum=w797, error in=w798) -> (error out=w791:errorcluster)  [unwired: 1 out]
        n380 = Merge Errors(w792, w791) -> (w790:errorcluster)
        n381 = call <vilib>:"Add State(s) to Queue__JKI_lib_State_Machine.vi"("State(s) in (\"\")"=w803) -> ("States Out"=w802:string)  [unwired: 14 in]
      }
    }
  }
